vi "9_3_2_8 Control_Signal_Test_Set SW3 OFF_R.vi"(11 "VariantIn":variant caption="Test Config Cluster Variant In") -> (0 "System Error Out":errorcluster, 3 "variantOut":variant caption="Test Config Cluster V ariant Out")   [LabVIEW 2020]
uses:
  <vilib>/Utility/miscctls.llb/LVRowAndColumnTypeDef.ctl
  <userlib>/_ATMF/Tools/Control/__TEST__SEQ__VARIABLES__.ctl
  <userlib>/_ATMF/Tools/Control/__STEP__DATA__.ctl
  <userlib>/_ATMF/Tools/Control/__STEP__DATA__TYPE__.ctl
  <userlib>/_ATMF/Tools/Control/__STEP__DATA__STATUS__TYPE__.ctl
  <userlib>/_ATMF/Tools/Control/__TEST__SEQ__CONFIG__CLUSTER__.ctl
  <userlib>/_ATMF/Control_Typedef/__TEST__STEP__VAR__UI__EXEC__MODE__.ctl
  <vilib>/Utility/miscctls.llb/LVBoundsTypeDef.ctl
  <vilib>/Utility/miscctls.llb/LVPositionTypeDef.ctl
  <userlib>/_ATMF/Tools/Control/__TABLE__ACTION__.ctl
  subvi/DM3058 Function Choose.ctl
  subvi/DCDC_Command.ctl
  70cdd13f-c836-49cb-97c4-706e2b611909.vi
  259f7c0d-0f00-4e2c-849c-bbf7e935248c.vi
  <vilib>/Utility/file.llb/Write Delimited Spreadsheet (string).vi
  <vilib>/Utility/file.llb/Read Delimited Spreadsheet (string).vi
  <userlib>/_ATMF/Tools/SubVIs/SubPalette_Update_Sequencer_Variable/SEQ.Update_Seq_Var_Module.Action.vi
  <userlib>/_ATMF/Tools/SubVIs/SubPalette_Update_Sequencer_Variable/SEQ.Update_Seq_Var_Module.Pass_Fail_Test.vi
  <userlib>/_ATMF/Tools/SubVIs/SubPalette_Update_Sequencer_Variable/Set_Max_Min/SEQ.Update_Seq_Var_Module.Set_Max_Min.vi
  <userlib>/_ATMF/Tools/SubVIs/SubPalette_Update_Sequencer_Variable/SEQ.Update_Seq_Var_Module.Numericl_Test.vi
  <vilib>/Comparison/Equal/Equal Functor/Equal Functor.lvclass
  <vilib>/addons/_JKI.lib/Serialization/JSON/JKI JSON Serialization.lvlib
  a62a6993-2855-4a98-a1d5-fd509ee8ed4e.vi
  fb335dba-24a3-4358-828e-e0ecb5c05990.vi
panel:
  in  "Instrument Serial":T1
  out "Cell Position":T2
  in  "stepsRing":u16(ring) items=["Next", "End", "--------------", "init", "Measure VPS1", "Measure VPS2", "Measure VPS3"]
  in  "exitButton":bool
  in  "saveButton":bool
  in  "runButton":bool
  in  "currentRetest":u8
  in  "totalSeqIndex":i32
  in  "currenIndex":i32
  in  "seqData[](Process)":string[][](array[string])
  in  "disMsg":refnum<vi>
  in  "seqData[](Original)":string[][](array[string])
  in  "Tab Control":enum32{"Sequence", "Input", "Output"}(tab)
  in  "stepName":string
  in  "Sequence List":i32[](listbox)=[0]
  in  "seqFilePath":path caption="Sequence File Path :"
  in  "userDef":T3={"VSP1 Min"=13.0, "VSP1 Max"=11.0, "VSP2 Min"=13.0, "VSP3 Max"=11.0, "VSP3 Min"=13.0, "VSP2 Max"=11.0, "L1 Min"=1.164, "L1 Max"=1.236, "L3 Min"=1.164, "L3 Max"=1.236, "D5 Min"=1.164, "D5 Max"=1.236, "D6 Min"=1.164, "D6 Max"=1.236, "D3 Min"=0.873, "D3 Max"=0.927, "D8 Min"=1.164, "D8 Max"=1.236, "APOS Max "=0.5, "ANEG Max"=-0.5, "DPOS Max"=0.5, "APOS Min"=0.5, "ANEG Min"=-0.5, "DPOS Min"=0.5} caption="User Input ( Save by Run Ctrl+R and click \"Save\" button  )"
  in  "varFilePath":path caption="Variable File Path :"
  in  "criteriaINI":path caption="Criteria(.ini) Path :"
  in  "displayMsg":string caption="Display Message"
  in  "testTable":i32(listbox)=-1 caption="Connectivity Test"
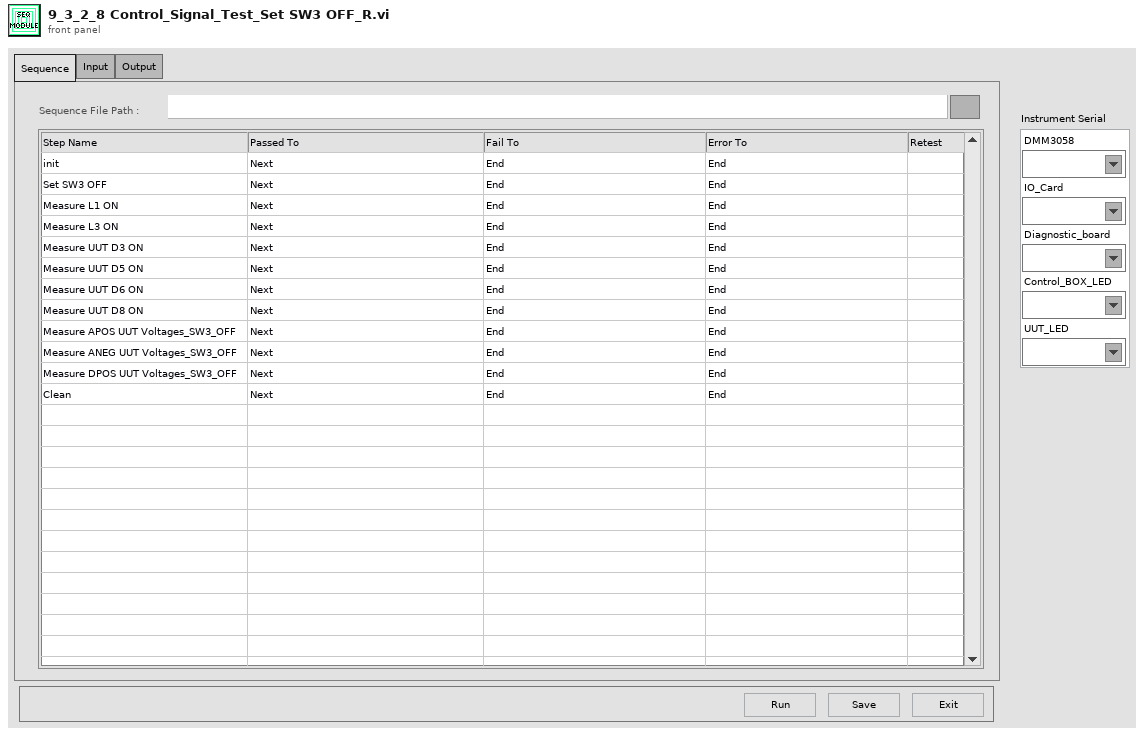
[diagram p1: front panel]
types:
  T1 = cluster{"DMM3058":refnum<visa-resource-name>, "IO_Card":refnum<visa-resource-name>, "Diagnostic_board":refnum<visa-resource-name>, "Control_BOX_LED":refnum<visa-resource-name>, "UUT_LED":refnum<visa-resource-name>}
  T2 = typedef "LVRowAndColumnTypeDef.ctl" = cluster{"Row":i32, "Column":i32}
  T3 = cluster{"VSP1 Min":dbl, "VSP1 Max":dbl, "VSP2 Min":dbl, "VSP3 Max":dbl, "VSP3 Min":dbl, "VSP2 Max":dbl, "L1 Min":dbl, "L1 Max":dbl, "L3 Min":dbl, "L3 Max":dbl, "D5 Min":dbl, "D5 Max":dbl, "D6 Min":dbl, "D6 Max":dbl, "D3 Min":dbl, "D3 Max":dbl, "D8 Min":dbl, "D8 Max":dbl, "APOS Max ":dbl, "ANEG Max":dbl, "DPOS Max":dbl, "APOS Min":dbl, "ANEG Min":dbl, "DPOS Min":dbl}
  T4 = typedef "__TEST__SEQ__VARIABLES__.ctl" = cluster{"stepData":T5, "testConfigCluster":T8}
  T5 = typedef "__STEP__DATA__.ctl" = cluster{"stepType":T6, "stepName":string, "description":string, "min":string, "measure":string, "max":string, "unit":string, "statusType":T7, "runMode":enum16{"Normal", "Skip"}, "viPath":path, "uutError":errorcluster, "passTo":string, "failTo":string, "errorTo":string, "parameter":string, "value":variant, "startTime":timestamp, "intervalLoop":u8, "retest":u8}
  T6 = typedef "__STEP__DATA__TYPE__.ctl" = enum16{"Action", "Pass/Fail Test", "Numeric Limit Test", "String Value Test"}
  T7 = typedef "__STEP__DATA__STATUS__TYPE__.ctl" = enum16{"DONE", "PASS", "FAIL", "ERROR", "SKIPPED"}
  T8 = typedef "__TEST__SEQ__CONFIG__CLUSTER__.ctl" = cluster{"slotIndex":u8, "execMode":T9, "mainConfigFile":path, "criteriaINI":path, "totalResult":bool, "stopIfFail":bool, "userControls":cluster{"dialog":refnum<vi>, "testTable":refnum<vi>, "stopButton":refnum<vi>, "statusBox":refnum<vi>}, "testedResult":enum16{"DONE", "PASS", "FAIL", "ERROR", "SKIPPED"}, "timeStamp":cluster{"Start":timestamp, "End":timestamp}, "repeatNum":u8, "uutInfo":cluster{"s/n":string, "p/n":string, "productRev":string}, "sysLanguage":enum16{"English", "Chinese", "Thai"}, "numOfSocket#":u8, "testRef":string, "testInfo":cluster{"testTime":string, "userID":string, "stationName":string, "testerID":string, "hwVer":string, "swVer":string, "fixtureID":string}}
  T9 = typedef "__TEST__STEP__VAR__UI__EXEC__MODE__.ctl" = enum16{"Run", "Debug", "Edit", "Open VI"}
  T10 = enum16{"open", "replace", "create", "open or create", "replace or create", "replace or create with confirmation"}
  T11 = typedef "LVPositionTypeDef.ctl" = cluster{"Left":i32, "Top":i32}
  T12 = typedef "LVBoundsTypeDef.ctl" = cluster{"Width":u32, "Height":u32}
  T13 = enum32{"Bad", "Idle", "Run top level", "Running"}
  T14 = typedef "__TABLE__ACTION__.ctl" = enum16{"Initial", "Append", "Clear", "Header"}
  T15 = enum16{"StepName", "PassTo", "FailTo", "ErrorTo", "Re-test"}
  T16 = enum16{"StepName", "PassTo", "FailTo", "ErrorTo"}
  T17 = cluster{"Reset (True)":bool, "ID Query (True)":bool, "Auto Range (T:Enable)":bool, "Function (0: DC Volts)":u16, "Range Select":enum16{"200mV", "2V", "20V", "200V", "1000V"}, "Absolute Resolution (0: 5.5 Rate:Slow)":u16}
  T18 = typedef "DM3058 Function Choose.ctl" = enum16{"Close", "Measure", "Config", "Init"}
  T19 = typedef "DCDC_Command.ctl" = enum16{"Reset", "APOS_SENSE", "ANEG_SENSE", "DPOS_SENSE", "FCT_SW1", "FCT_SW2", "FCT_SW3", "ANEG_LOAD", "APOS_LOAD", "DPOS_LOAD", "Short ANEG", "Short APOS", "Short DPOS", "meas_PSU_1_12V", "meas_PSU_2_12V", "meas_PSU_3_12V", "meas_UUT_APOS_voltage", "meas_UUT_ANEG_voltage", "meas_UUT_DPOS_voltage", "meas_LOAD_APOS_voltage", "meas_LOAD_ANEG_voltage", "meas_LOAD_DPOS_voltage", "UUT_FCT_power_SW", "Burn_in_FAN_SW", "FCT_FAN_SW", "FCT_24V_SW", "USB_Reset", "DMM_SW"}
  T20 = typedef "LVPoint32TypeDef.ctl" = cluster{"Horizontal":i32, "Vertical":i32}
  T21 = typedef "LVFontTypeDef.ctl" = cluster{"Font Name":string, "Size":u16, "Bold":bool, "Italic":bool, "Underline":bool, "Strikeout":bool, "Color":u32}
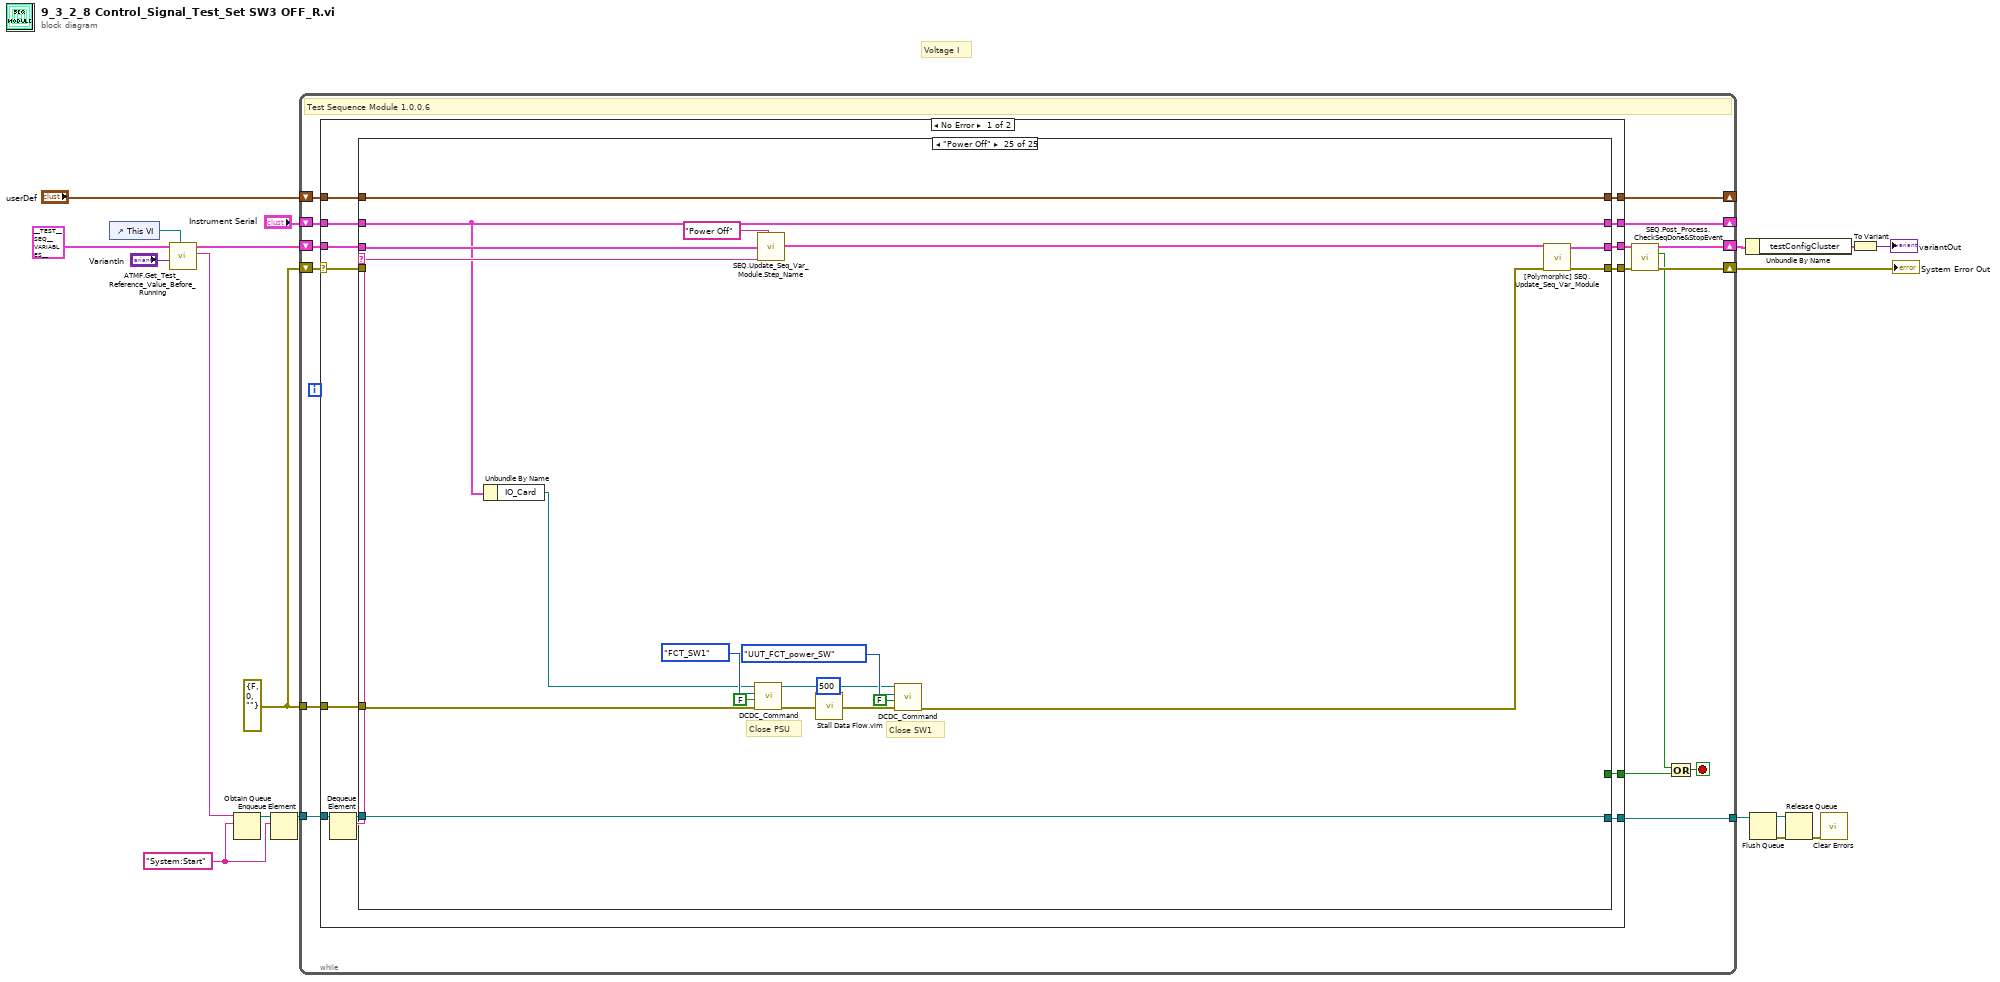
[diagram p0: block diagram]
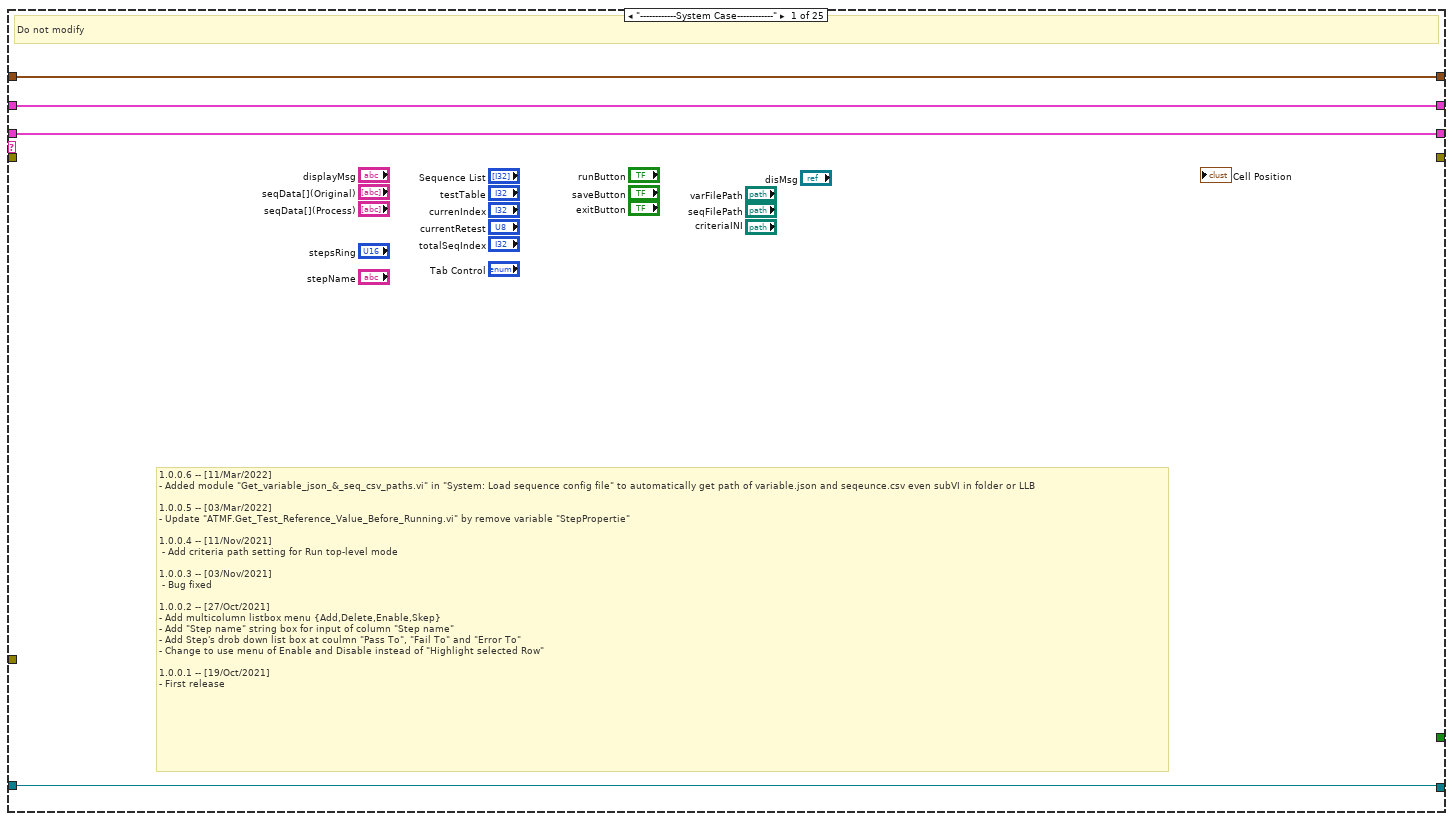
[diagram p2: hidden frame]
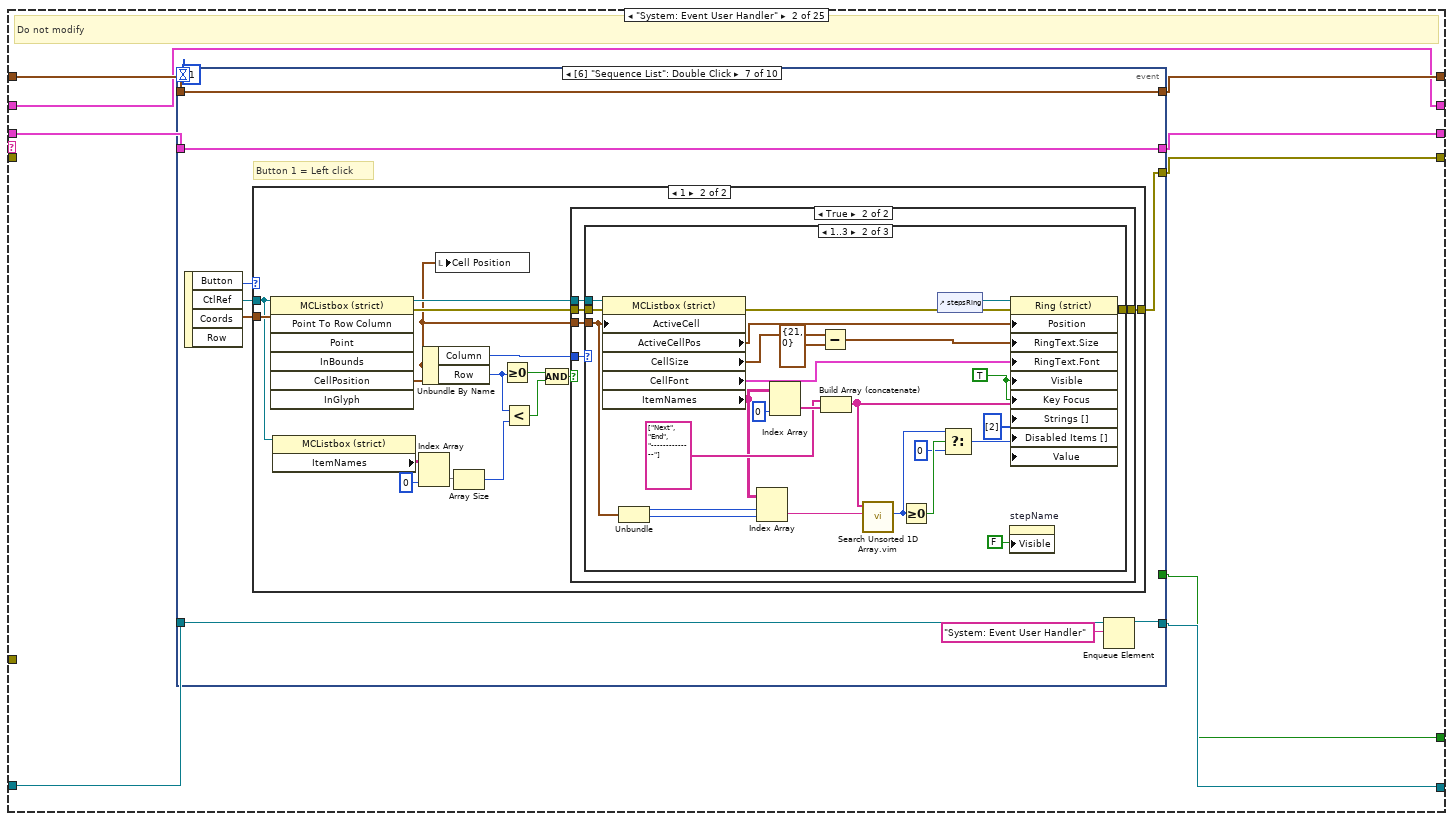
[diagram p3: hidden frame]
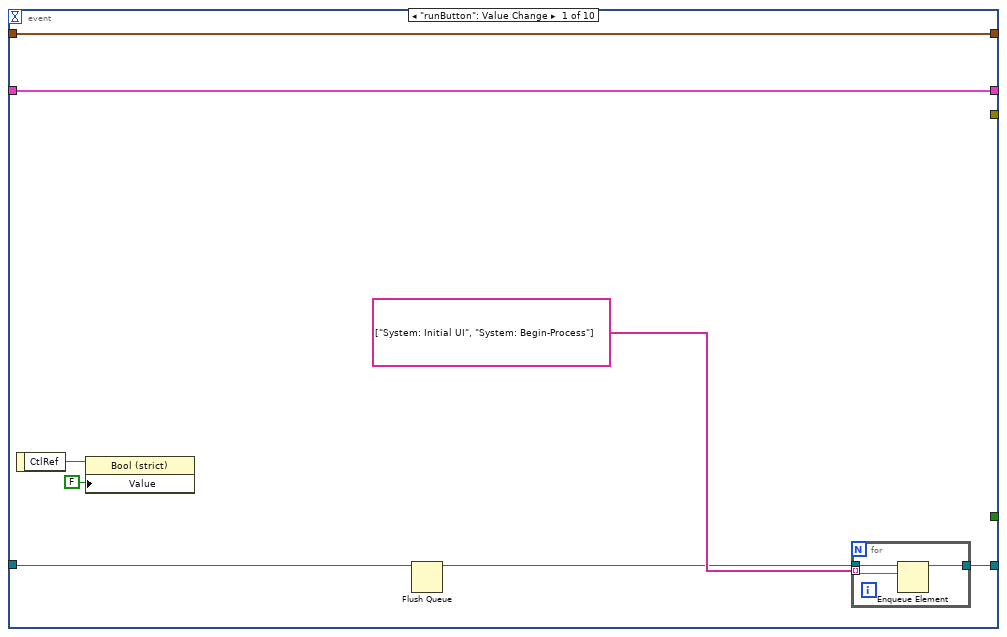
[diagram p4: hidden frame]
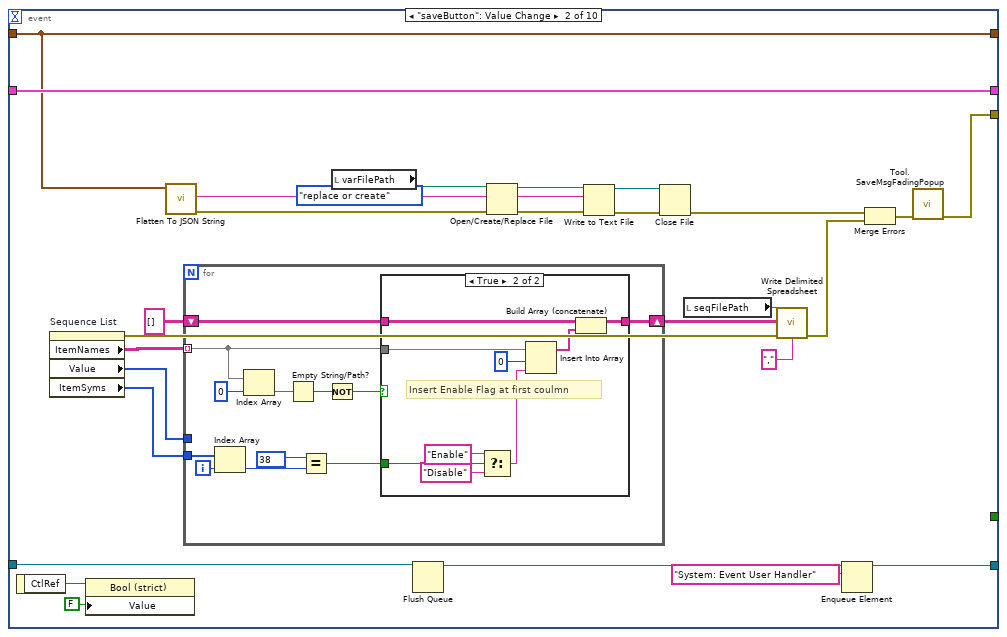
[diagram p5: hidden frame]
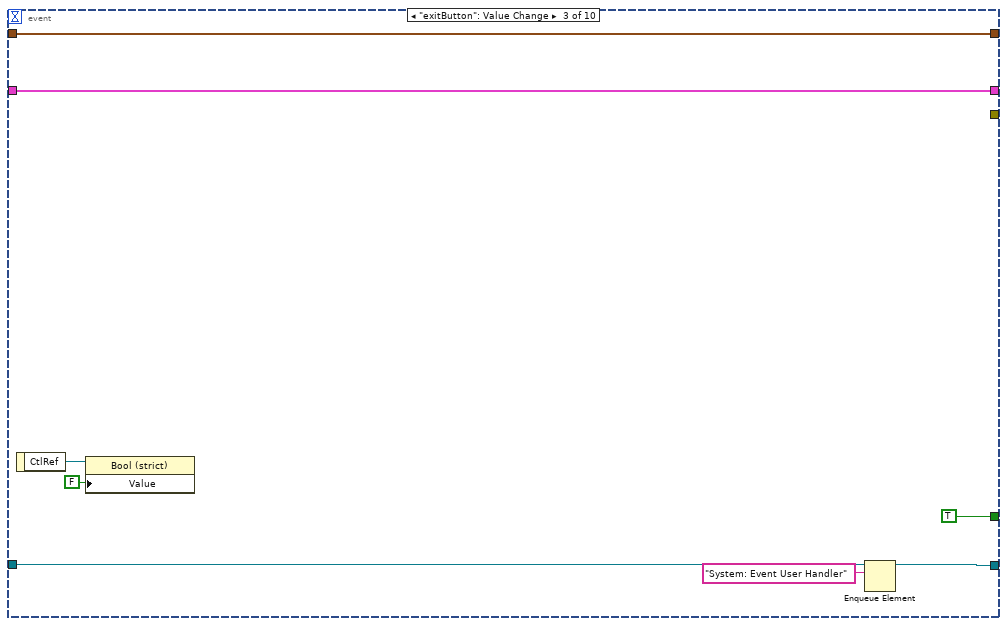
[diagram p7: hidden frame]
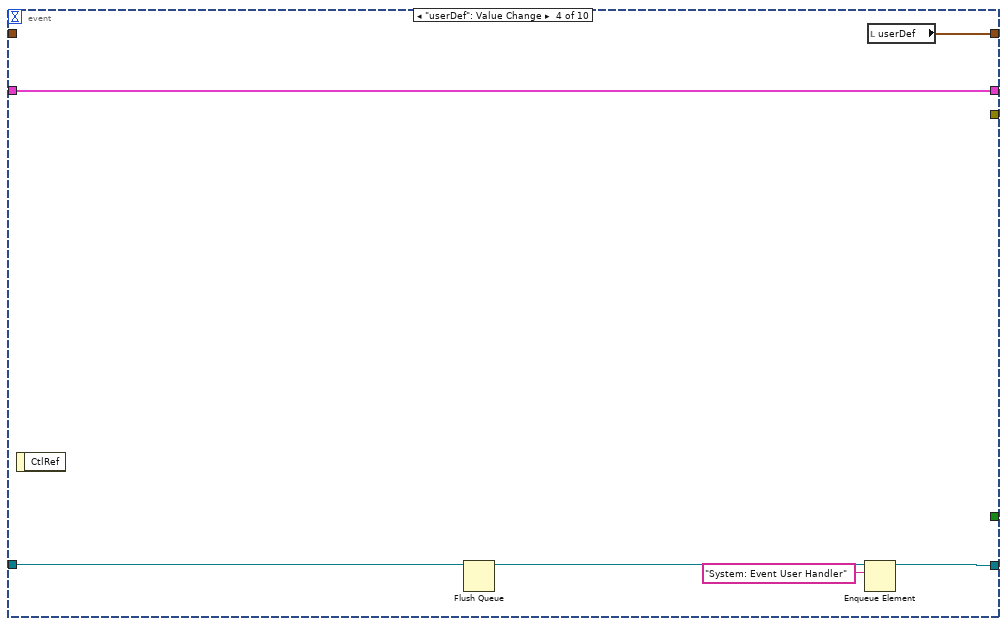
[diagram p8: hidden frame]
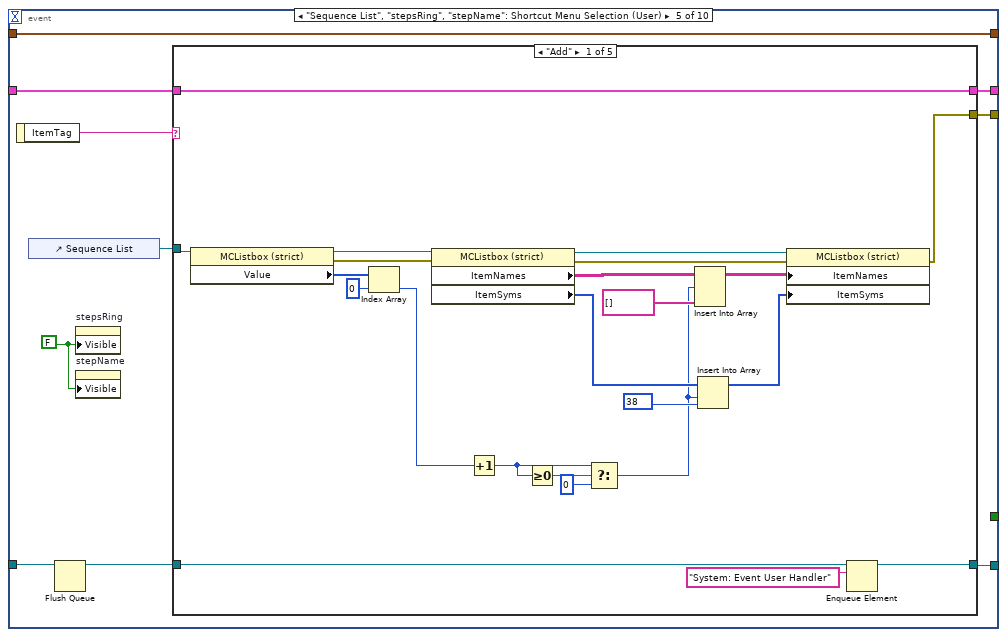
[diagram p9: hidden frame]
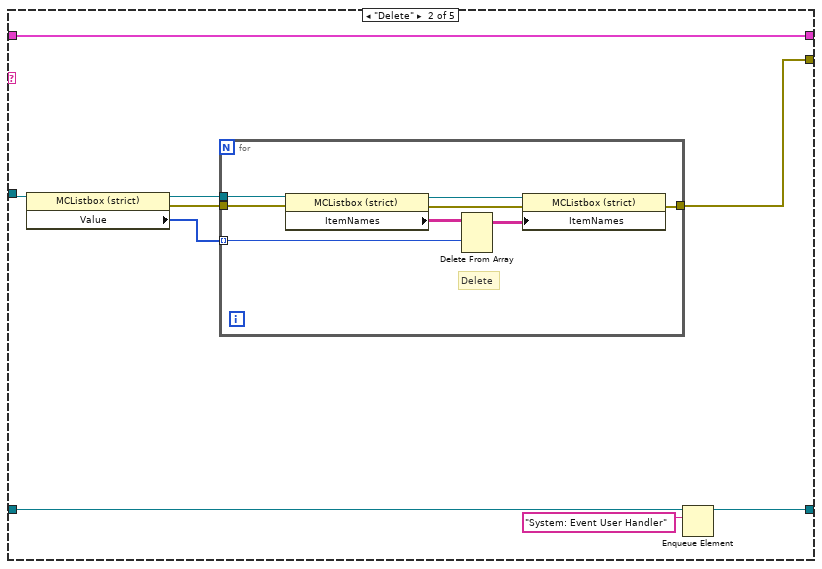
[diagram p10: hidden frame]
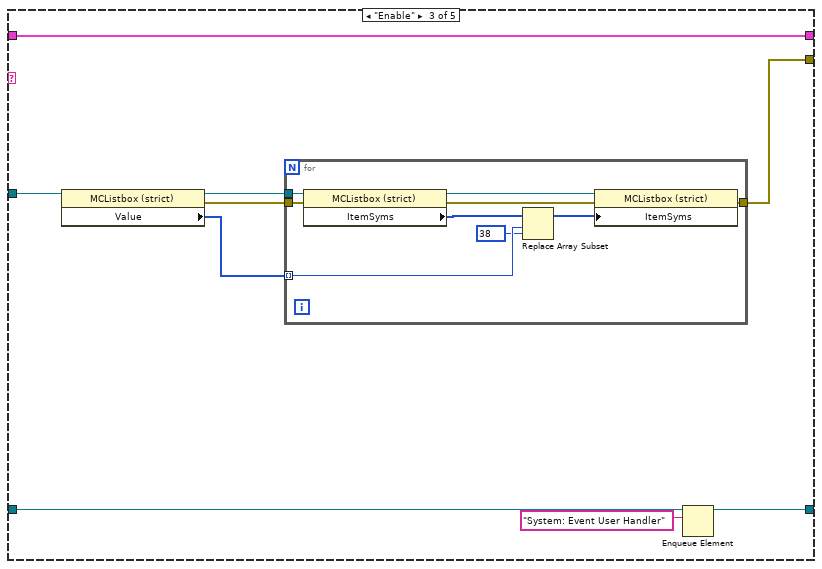
[diagram p11: hidden frame]
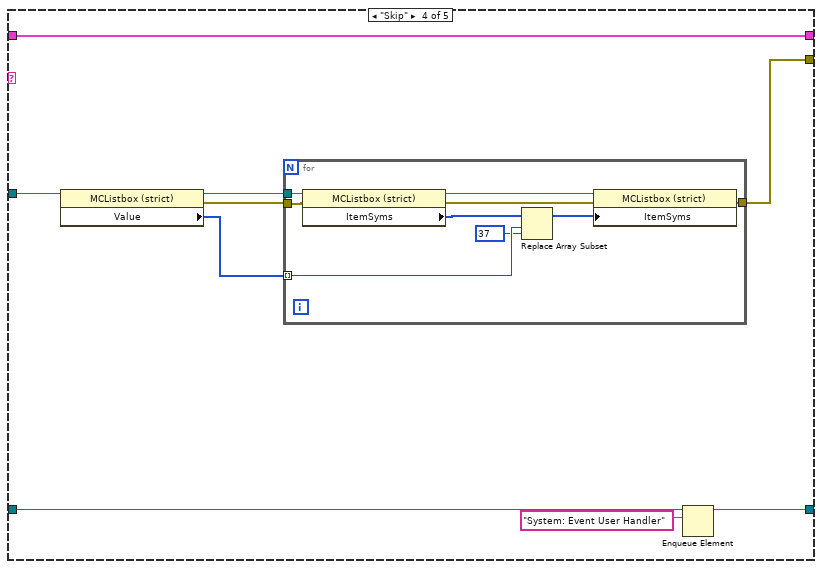
[diagram p12: hidden frame]
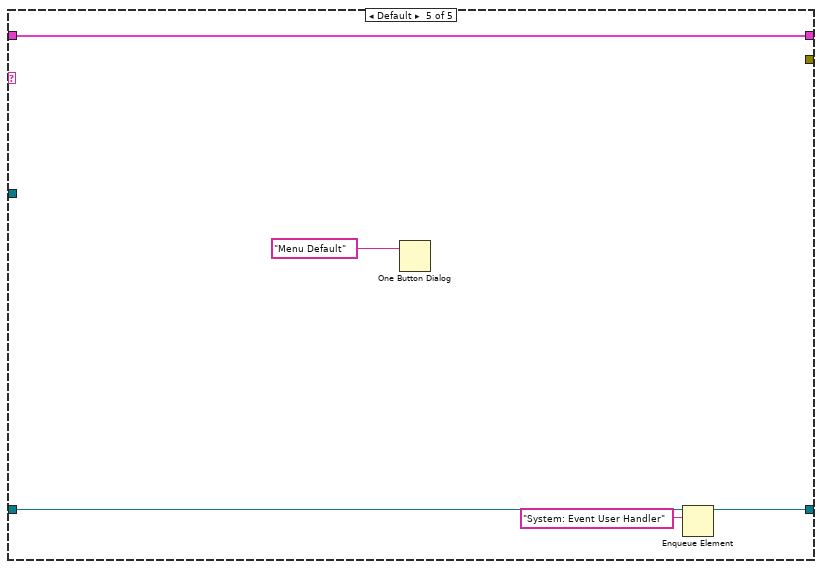
[diagram p13: hidden frame]
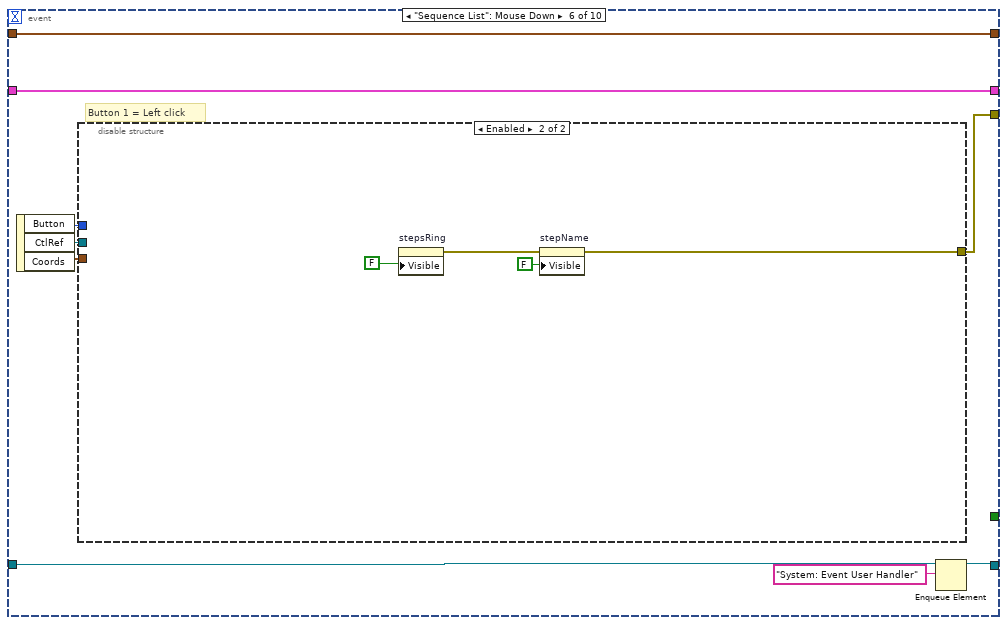
[diagram p14: hidden frame]
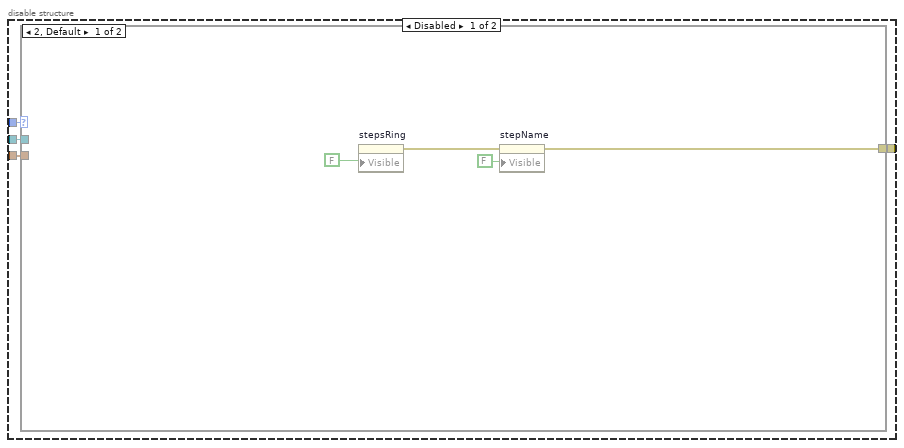
[diagram p15: hidden frame]
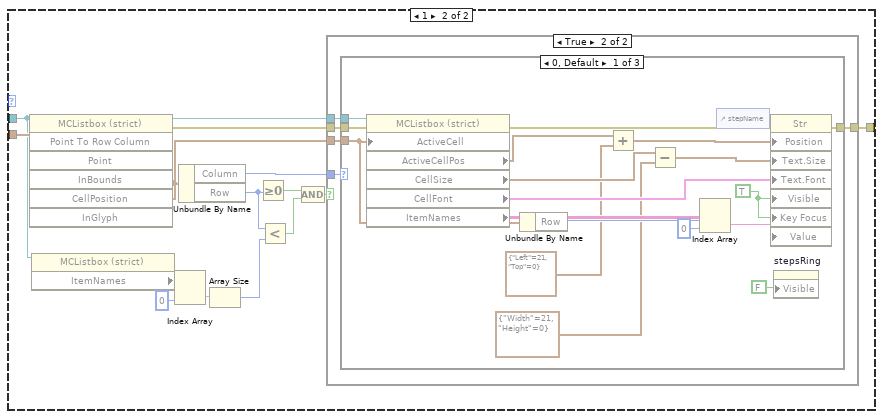
[diagram p16: hidden frame]
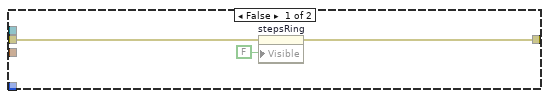
[diagram p17: hidden frame]
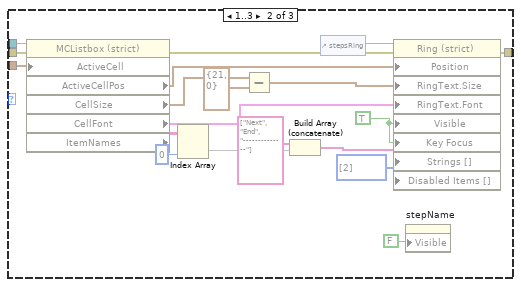
[diagram p18: hidden frame]
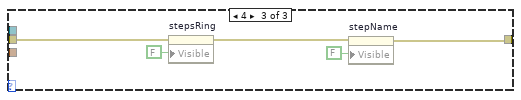
[diagram p19: hidden frame]
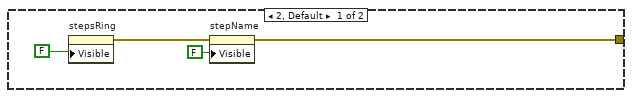
[diagram p20: hidden frame]
diagram:
  w2 = errorcluster {"status"=FALSE, "code"=0, "source"=""} ("UUT Error In")
  w14 = "System:Start"
  # "Voltage I"
  n1 = control-ref of="This VI"() -> (w6:refnum<vi>)
  n2 = call <userlib>:"ATMF.Get_Test_Reference_Value_Before_Running.vi"("viRef"=w6, "Variant"="VariantIn", "seqDataIn"=T4 {"stepData"={"stepType"=enum."Action", "stepName"="", "description"="", "min"="", "measure"="", "max"="", "unit"="", "statusType"=enum."DONE", "runMode"=enum."Normal", "viPath"=path "", "uutError"={"status"=FALSE, "code"=0, "source"=""}, "passTo"="", "failTo"="", "errorTo"="", "parameter"="", "value"=variant(string[][] []), "startTime"=timestamp(0 s since 1904-01-01), "intervalLoop"=1, "retest"=0}, "testConfigCluster"={"slotIndex"=0, "execMode"=enum."Run", "mainConfigFile"=path "", "criteriaINI"=path "", "totalResult"=FALSE, "stopIfFail"=FALSE, "userControls"={"dialog"=refnum, "testTable"=refnum, "stopButton"=refnum, "statusBox"=refnum}, "testedResult"=enum."DONE", "timeStamp"={"Start"=timestamp(0 s since 1904-01-01), "End"=timestamp(0 s since 1904-01-01)}, "repeatNum"=1, "uutInfo"={"s/n"="", "p/n"="", "productRev"=""}, "sysLanguage"=enum."English", "numOfSocket#"=1, "testRef"="", "testInfo"={"testTime"="", "userID"="", "stationName"="", "testerID"="", "hwVer"="", "swVer"="", "fixtureID"=""}}} ("localVar")) -> ("testRef#"=w9:string, "seqDataOut"=w7:T4)  [unwired: 6 in, 1 out]
  n3 = Obtain Queue(name (unnamed)=w9, element data type=w14) -> (queue out=w19:refnum<queue>)  [unwired: 3 in, 2 out]
  n4 = Enqueue Element(queue=w19, element=w14) -> (queue out=w17:refnum<queue>)  [unwired: 2 in, 2 out]
  n5 = while {
    shift-right: [w25] -> w11
    shift-left: w2 -> [w35]
    shift-right: [w27] -> w5
    shift-left: w7 -> [w34]
    tunnel: w17 -> [w33]
    tunnel: [w32] -> w16
    tunnel: w2 -> [w30]
    shift-right: [w29] -> _
    shift-left: "userDef" -> [w31]
    shift-right: [w21] -> _
    shift-left: "Instrument Serial" -> [w20]
    stop <- w22 stop-if-true
    # "Test Sequence Module 1.0.0.6"
    n6 = case shown="No Error" w35 {
      selector: w35 -> [w47 w1153]
      tunnel: [w46 w1153] -> w26
      tunnel: w34 -> [w49 w1160]
      tunnel: [w48 w1160] -> w28
      tunnel: [w45 TRUE] -> w23
      tunnel: [w42 w1158] -> w32
      tunnel: w33 -> [w41 w1155]
      tunnel: w31 -> [w39 w1154]
      tunnel: w30 -> [w40 _]
      tunnel: [w38 w1154] -> w29
      tunnel: [w37 w1152] -> w21
      tunnel: w20 -> [w36 w1152]
      frame No Error {
        n7 = Dequeue Element(queue=w41) -> (queue out=w43:refnum<queue>, element=w44:string)  [unwired: 2 in, 2 out]
        n8 = case shown="\"Power Off\"" w44 {
          selector: w44 -> [_ _ _ _ _ _ _ _ _ _ _ w763 _ w776 w820 w843 w866 w890 w912 w935 w959 w981 w1036 w1089 w1149]
          tunnel: w49 -> [w52 w60 w438 w472 w484 w535 w622 w638 w683 w707 w740 w767 w770 w814 w821 w855 w878 w901 w924 w947 w970 w996 w1050 w1104 w1148]
          tunnel: [w52 w59 w440 w475 w493 w535 w622 w640 w682 w715 w743 w767 w770 w813 w818 w854 w877 w900 w923 w946 w969 w993 w1047 w1101 w1144] -> w48
          tunnel: w47 -> [_ _ _ _ _ _ _ _ _ _ _ _ _ w775 w819 w844 w871 w889 w917 w940 w958 w982 w1035 w1091 _]
          tunnel: [_ w55 _ _ w494 w533 _ _ _ _ _ w759 _ w812 w817 w853 w876 w899 w922 w945 w968 w994 w1048 w1102 w1145] -> w46
          tunnel: [_ w56 _ _ _ _ _ _ _ _ w746 TRUE _ _ _ _ _ _ _ _ _ _ _ _ _] -> w45
          tunnel: w43 -> [w51 w63 w450 w473 w491 w536 w628 w642 w681 w714 w742 w765 w769 w811 _ w852 w875 w898 w921 w944 w967 w997 w1051 w1105 w1146]
          tunnel: [w51 w58 w449 w473 w490 w536 w627 w641 w680 w713 w741 w765 w769 w811 _ w852 w875 w898 w921 w944 w967 w997 w1051 w1105 w1146] -> w42
          tunnel: w40 -> [_ _ _ _ _ _ _ _ _ _ _ _ _ w790 w824 w842 w863 w885 w909 w931 w955 w990 w1044 w1100 w1141]
          tunnel: w39 -> [w53 w62 w442 w474 w495 w532 w617 w639 w685 w716 w745 w764 w771 w809 w823 w851 w874 w897 w920 w943 w966 w988 w1042 w1096 w1147]
          tunnel: [w53 w61 w441 w474 w495 w531 w617 w639 w685 w716 w744 w764 w771 w809 w823 w851 w874 w897 w920 w943 w966 w988 w1042 w1096 w1147] -> w38
          tunnel: [w50 w54 w436 w470 w483 w526 w616 w629 w679 w705 w738 w757 w768 w781 w822 w849 w872 w895 w918 w941 w964 w992 w1043 w1098 w1134] -> w37
          tunnel: w36 -> [w50 w54 w436 w470 w483 w526 w616 w629 w679 w705 w738 w757 w768 w808 w822 w849 w872 w895 w918 w941 w964 w992 w1043 w1098 w1134]
          frame "------------System Case------------" {
            # "1.0.0.6 -- [11/Mar/2022]\n- Added module \"Get_variable_json_&_seq_csv_paths.vi\" in \"System: Load sequence config file\" to automatically get path of variable.json and seqeunce.csv even subVI in folder or LLB\n\n1.0.0.5 -- [03/Mar/2022]\n- Update \"ATMF.Get_Test_Reference_Value_Before_Running.vi\" by remove variable \"StepPropertie\"\n\n1.0.0.4 -- [11/Nov/2021]\n - Add criteria path setting for Run top-level mode\n\n1.0.0.3 -- [03/Nov/2021]\n - Bug fixed \n\n1.0.0.2 -- [27/Oct/2021]\n- Add multicolumn listbox menu {Add,Delete,Enable,Skep}\n- Add \"Step name\" string box for input of column \"Step name\"\n- Add Step's drob down list box at coulmn \"Pass To\", \"Fail To\" and \"Error To\"\n- Change to use menu of Enable and Disable instead of \"Highlight selected Row\"\n\n1.0.0.1 -- [19/Oct/2021]\n- First release"
            # "Do not modify"
          }
          frame "System: Event User Handler" {
            # "Do not modify"
            n9 = event shown="[6] \"Sequence List\": Double Click" {
              selector: _ -> [_ _ _ _ _ _ _ _ _ _]
              dyn-events: _ -> [_ _ _ _ _ _ _ _ _ _]
              timeout: -1 -> [_ _ _ _ _ _ _ _ _ _]
              tunnel: w63 -> [w64 w86 w126 w133 w142 w236 w323 w404 w424 w433]
              tunnel: w62 -> [w71 w99 w132 _ w147 w238 w325 w415 w432 w435]
              tunnel: [w71 w99 w132 w135 w147 w238 w325 w415 w432 w435] -> w61
              tunnel: w60 -> [w70 w102 w131 w138 w145 w237 w324 w414 w431 w434]
              tunnel: [w70 w102 w131 w138 w146 w237 w324 w414 w431 w434] -> w59
              tunnel: [w69 w89 w127 w137 w148 w235 w322 w405 w425 w433] -> w58
              tunnel: [_ _ TRUE _ _ _ _ _ _ _] -> w56
              tunnel: [_ w97 _ _ w141 w231 w318 w411 w428 _] -> w55
              event "runButton": Value Change {
                n10 = event-data() -> ("CtlRef"=w68:refnum<vi>)  [unwired: 1 in]
                n11 = property class="Bool (strict)"(reference=w68, "Value"=FALSE) -> ()  [unwired: 1 in, 2 out]
                n12 = Flush Queue(queue=w64) -> (queue out=w65:refnum<queue>)  [unwired: 1 in, 2 out]
                n13 = for {
                  tunnel: w65 -> [w74]
                  tunnel: [w73] -> w69
                  tunnel: string[] ["System: Initial UI", "System: Begin-Process"] -> [w72] mode=indexing
                  n14 = Enqueue Element(queue=w74, element=w72) -> (queue out=w73:refnum<queue>)  [unwired: 2 in, 2 out]
                }
              }
              event "saveButton": Value Change {
                n15 = event-data() -> ("CtlRef"=w101:refnum<vi>)  [unwired: 1 in]
                n16 = property on="Sequence List" class="MCListbox (strict)"() -> (error out=w85:errorcluster, "ItemNames"=w81:string[][], "Value"=w82:i32[], "ItemSyms"=w75:i32[])  [unwired: 2 in, 1 out]
                n17 = property class="Bool (strict)"(reference=w101, "Value"=FALSE) -> ()  [unwired: 1 in, 2 out]
                n18 = call <vilib>:"Flatten To JSON String.vi"("Variant"=w99) -> ("error out"=w98:errorcluster, "JSON String"=w91:string)  [unwired: 9 in]
                n19 = for {
                  tunnel: w82 -> [_]
                  tunnel: w81 -> [w112] mode=indexing
                  shift-right: [w108] -> w79
                  shift-left: string[][] [] -> [w109]
                  tunnel: w75 -> [w107]
                  i -> [w106]
                  n20 = Index Array(array=w107, index=w106) -> (element=w105:i32)
                  n21 = Index Array(array=w112, index=0) -> (element=w110:string)
                  n22 = Empty String/Path?(string/path=w110) -> (empty?=w114:bool)
                  n23 = Equal?(x=38, y=w105) -> (x = y?=w103:bool)
                  n24 = Not(x=w114) -> (.not. x?=w113:bool)
                  n25 = case shown="True" w113 {
                    tunnel: w112 -> [_ w124]
                    tunnel: w109 -> [w115 w120]
                    tunnel: [w115 w119] -> w108
                    tunnel: w103 -> [_ w116]
                    frame False {
                    }
                    frame True {
                      # "Insert Enable Flag at first coulmn"
                      n26 = Select(t="Enable", s=w116, f="Disable") -> (s? t:f=w121:string)
                      n27 = Insert Into Array(array=w124, index=0, new element=w121) -> (w118:string[])
                      n28 = Build Array (concatenate)(w120, w118) -> (w119:string[][])
                    }
                  }
                }
                n29 = local read "varFilePath"() -> (w92:path)
                n30 = Flush Queue(queue=w86) -> (queue out=w87:refnum<queue>)  [unwired: 1 in, 2 out]
                n31 = Open/Create/Replace File(file path (use dialog)=w92, error in=w98, operation (0:open)=T10."replace or create") -> (refnum out=w94:refnum<file>, error out=w96:errorcluster)  [unwired: 3 in, 1 out]
                n32 = Write to Text File(file (use dialog)=w94, text=w91, error in=w96) -> (refnum out=w93:refnum<file>, error out=w95:errorcluster)  [unwired: 1 in, 1 out]
                n33 = Close File(refnum=w93, error in=w95) -> (error out=w77:errorcluster)  [unwired: 1 out]
                n34 = local read "seqFilePath"() -> (w83:path)
                n35 = call-poly <vilib>:"Write Delimited Spreadsheet.vi"("file path (dialog if empty)"=w83, "2D data"=w79, "error in (no error)"=w85, "delimiter (\\t)"="," ("delimiter (\\t)")) -> ("error out"=w78:errorcluster)  [unwired: 10 in, 1 out]
                n36 = Enqueue Element(queue=w87, element="System: Event User Handler") -> (queue out=w89:refnum<queue>)  [unwired: 2 in, 2 out]
                n37 = Merge Errors(w77, w78) -> (w76:errorcluster)
                n38 = call <userlib>:"Tool.SaveMsgFadingPopup.vi"("error in"=w76) -> ("error out"=w97:errorcluster)  [unwired: 10 in]
              }
              event "exitButton": Value Change {
                n39 = event-data() -> ("CtlRef"=w130:refnum<vi>)  [unwired: 1 in]
                n40 = property class="Bool (strict)"(reference=w130, "Value"=FALSE) -> ()  [unwired: 1 in, 2 out]
                n41 = Enqueue Element(queue=w126, element="System: Event User Handler") -> (queue out=w127:refnum<queue>)  [unwired: 2 in, 2 out]
              }
              event "userDef": Value Change {
                n42 = event-data() -> ()  [unwired: 1 in, 1 out]
                n43 = Flush Queue(queue=w133) -> (queue out=w134:refnum<queue>)  [unwired: 1 in, 2 out]
                n44 = Enqueue Element(queue=w134, element="System: Event User Handler") -> (queue out=w137:refnum<queue>)  [unwired: 2 in, 2 out]
                n45 = local read "userDef"() -> (w135:T3)
              }
              event "Sequence List", "stepsRing", "stepName": Shortcut Menu Selection (User) {
                w139 = FALSE
                n46 = event-data() -> ("ItemTag"=w144:string)  [unwired: 1 in]
                n47 = control-ref of="Sequence List"() -> (w140:refnum<vi>)
                n48 = Flush Queue(queue=w142) -> (queue out=w143:refnum<queue>)  [unwired: 1 in, 2 out]
                n49 = property on="stepsRing" class="Ring (strict)"("Visible"=w139) -> ()  [unwired: 2 in, 2 out]
                n50 = property on="stepName" class="Str"("Visible"=w139) -> ()  [unwired: 2 in, 2 out]
                n51 = case shown="\"Add\"" w144 {
                  tunnel: [w171 w180 w197 w215 w229] -> w148
                  tunnel: w143 -> [w169 w178 w195 w213 w227]
                  tunnel: [w168 w177 w194 w212 w226] -> w146
                  tunnel: w145 -> [w168 w177 w194 w212 w226]
                  tunnel: w140 -> [w149 w173 w193 w211 _]
                  tunnel: [w161 w174 w189 w207 _] -> w141
                  frame "Add" {
                    n52 = property class="MCListbox (strict)"(reference=w149) -> (reference out=w165:refnum<vi>, error out=w164:errorcluster, "Value"=w167:i32[])  [unwired: 1 in]
                    n53 = Index Array(array=w167, index=0) -> (element=w152:i32)
                    n54 = property class="MCListbox (strict)"(reference=w165, error in=w164) -> (reference out=w163:refnum<vi>, error out=w162:errorcluster, "ItemNames"=w160:string[][], "ItemSyms"=w157:i32[])
                    n55 = Increment(x=w152) -> (x+1=w154:i32)
                    n56 = Greater Or Equal To 0?(x=w154) -> (x >= 0?=w153:bool)
                    n57 = Select(t=w154, s=w153, f=0) -> (s? t:f=w151:i32)
                    n58 = Insert Into Array(array=w160, index (row)=w151, new element=string[] [] ("new element/subarray")) -> (w159:string[][])  [unwired: 1 in]
                    n59 = Insert Into Array(array=w157, index=w151, new element=38) -> (w155:i32[])
                    n60 = property class="MCListbox (strict)"(reference=w163, error in=w162, "ItemNames"=w159, "ItemSyms"=w155) -> (error out=w161:errorcluster)  [unwired: 1 out]
                    n61 = Enqueue Element(queue=w169, element="System: Event User Handler") -> (queue out=w171:refnum<queue>)  [unwired: 2 in, 2 out]
                  }
                  frame "Delete" {
                    n62 = property class="MCListbox (strict)"(reference=w173) -> (reference out=w176:refnum<vi>, error out=w175:errorcluster, "Value"=w172:i32[])  [unwired: 1 in]
                    n63 = for {
                      tunnel: w176 -> [w188]
                      tunnel: w175 -> [w187]
                      tunnel: [w184] -> w174
                      tunnel: w172 -> [w182] mode=indexing
                      # "Delete"
                      n64 = property class="MCListbox (strict)"(reference=w188, error in=w187) -> (reference out=w186:refnum<vi>, error out=w185:errorcluster, "ItemNames"=w183:string[][])
                      n65 = Delete From Array(array=w183, index (row)=w182) -> (array with subset deleted=w181:string[][])  [unwired: 2 in, 1 out]
                      n66 = property class="MCListbox (strict)"(reference=w186, error in=w185, "ItemNames"=w181) -> (error out=w184:errorcluster)  [unwired: 1 out]
                    }
                    n67 = Enqueue Element(queue=w178, element="System: Event User Handler") -> (queue out=w180:refnum<queue>)  [unwired: 2 in, 2 out]
                  }
                  frame "Enable" {
                    n68 = property class="MCListbox (strict)"(reference=w193) -> (reference out=w191:refnum<vi>, error out=w190:errorcluster, "Value"=w192:i32[])  [unwired: 1 in]
                    n69 = for {
                      tunnel: w192 -> [w202] mode=indexing
                      tunnel: w191 -> [w206]
                      tunnel: w190 -> [w200]
                      tunnel: [w198] -> w189
                      n70 = property class="MCListbox (strict)"(reference=w206, error in=w200) -> (reference out=w204:refnum<vi>, error out=w199:errorcluster, "ItemSyms"=w205:i32[])
                      n71 = Replace Array Subset(array=w205, new element=38, index=w202) -> (w203:i32[])
                      n72 = property class="MCListbox (strict)"(reference=w204, error in=w199, "ItemSyms"=w203) -> (error out=w198:errorcluster)  [unwired: 1 out]
                    }
                    n73 = Enqueue Element(queue=w195, element="System: Event User Handler") -> (queue out=w197:refnum<queue>)  [unwired: 2 in, 2 out]
                  }
                  frame "Skip" {
                    n74 = property class="MCListbox (strict)"(reference=w211) -> (reference out=w209:refnum<vi>, error out=w208:errorcluster, "Value"=w210:i32[])  [unwired: 1 in]
                    n75 = for {
                      tunnel: w210 -> [w220] mode=indexing
                      tunnel: w209 -> [w224]
                      tunnel: w208 -> [w218]
                      tunnel: [w216] -> w207
                      n76 = property class="MCListbox (strict)"(reference=w224, error in=w218) -> (reference out=w222:refnum<vi>, error out=w217:errorcluster, "ItemSyms"=w223:i32[])
                      n77 = Replace Array Subset(array=w223, new element=37, index=w220) -> (w221:i32[])
                      n78 = property class="MCListbox (strict)"(reference=w222, error in=w217, "ItemSyms"=w221) -> (error out=w216:errorcluster)  [unwired: 1 out]
                    }
                    n79 = Enqueue Element(queue=w213, element="System: Event User Handler") -> (queue out=w215:refnum<queue>)  [unwired: 2 in, 2 out]
                  }
                  frame Default {
                    n80 = One Button Dialog(message="Menu Default") -> ()  [unwired: 1 in, 1 out]
                    n81 = Enqueue Element(queue=w227, element="System: Event User Handler") -> (queue out=w229:refnum<queue>)  [unwired: 2 in, 2 out]
                  }
                }
              }
              event "Sequence List": Mouse Down {
                # "Button 1 = Left click"
                n82 = event-data() -> ("Button"=w230:u16, "CtlRef"=w232:refnum<vi>, "Coords"=w233:T20)  [unwired: 1 in]
                n83 = disable-structure shown="Enabled" {
                  disable-tunnel: w233 -> [w242 _]
                  disable-tunnel: w232 -> [w241 _]
                  disable-tunnel: [w240 w313] -> w231
                  disable-tunnel: w230 -> [w239 _]
                  frame Disabled {
                    n84 = case shown="2, Default" w239 {
                      tunnel: w242 -> [_ w261]
                      tunnel: w241 -> [_ w257]
                      tunnel: [w243 w247] -> w240
                      frame 2, Default {
                        n85 = property on="stepsRing" class="Ring (strict)"("Visible"=FALSE) -> (error out=w245:errorcluster)  [unwired: 2 in, 1 out]
                        n86 = property on="stepName" class="Str"(error in=w245, "Visible"=FALSE) -> (error out=w243:errorcluster)  [unwired: 1 in, 1 out]
                      }
                      frame 1 {
                        n87 = invoke class="MCListbox (strict)" method="Point To Row Column"(reference=w257, "Point"=w261) -> (reference out=w260:refnum<vi>, error out=w259:errorcluster, "CellPosition"=w258:T2)  [unwired: 5 in, 4 out]
                        n88 = property class="MCListbox (strict)"(reference=w257) -> ("ItemNames"=w256:string[][])  [unwired: 1 in, 2 out]
                        n89 = Index Array(array=w256, index (col)=0 ("disabled index (col)")) -> (element=w254:string[])  [unwired: 1 in]
                        n90 = Unbundle By Name(w258) -> ("Column"=w248:i32, "Row"=w251:i32)
                        n91 = Array Size(array=w254) -> (size(s)=w250:i32)
                        n92 = Greater Or Equal To 0?(x=w251) -> (x >= 0?=w253:bool)
                        n93 = Less?(x=w251, y=w250) -> (x < y?=w249:bool)
                        n94 = Compound Arithmetic op=AND(w253, w249) -> (w252:bool)
                        n95 = case shown="True" w252 {
                          tunnel: w260 -> [_ w269]
                          tunnel: w259 -> [w264 w268]
                          tunnel: w258 -> [_ w267]
                          tunnel: [w263 w266] -> w247
                          tunnel: w248 -> [_ w265]
                          frame False {
                            n96 = property on="stepsRing" class="Ring (strict)"(error in=w264, "Visible"=FALSE) -> (error out=w263:errorcluster)  [unwired: 1 in, 1 out]
                          }
                          frame True {
                            n97 = case shown="0, Default" w265 {
                              tunnel: w269 -> [w286 w307 _]
                              tunnel: w268 -> [w284 w306 w311]
                              tunnel: w267 -> [w281 w305 _]
                              tunnel: [w287 w291 w308] -> w266
                              frame 0, Default {
                                w276 = TRUE ("Visible")
                                n98 = property on="Property Node" class="MCListbox (strict)"(reference=w286, error in=w284, "ActiveCell"=w281) -> (error out=w285:errorcluster, "ActiveCellPos"=w272:T11, "CellSize"=w275:T12, "CellFont"=w283:T21, "ItemNames"=w282:string[][])  [unwired: 1 out]
                                n99 = Unbundle By Name(w281) -> ("Row"=w280:i32)
                                n100 = Add(x=w272, y=T11 {"Left"=21, "Top"=0}) -> (x+y=w271:T11)
                                n101 = Subtract(x=w275, y=T12 {"Width"=21, "Height"=0}) -> (x-y=w273:T12)
                                n102 = Index Array(array=w282, index (row)=w280, index (col)=0 ("disabled index (col)")) -> (element=w278:string)
                                n103 = control-ref of="stepName"() -> (w288:refnum<vi>)
                                n104 = property on="Property Node" class="Str"(reference=w288, error in=w285, "Position"=w271, "Text.Size"=w273, "Text.Font"=w283, "Visible"=w276, "Key Focus"=w276, "Value"=w278) -> (error out=w287:errorcluster)  [unwired: 1 out]
                                n105 = property on="stepsRing" class="Ring (strict)"("Visible"=FALSE) -> ()  [unwired: 2 in, 2 out]
                              }
                              frame 1..3 {
                                w297 = TRUE ("Visible")
                                n106 = property on="Property Node" class="MCListbox (strict)"(reference=w307, error in=w306, "ActiveCell"=w305) -> (error out=w304:errorcluster, "ActiveCellPos"=w302:T11, "CellSize"=w300:T12, "CellFont"=w301:T21, "ItemNames"=w296:string[][])  [unwired: 1 out]
                                n107 = Index Array(array=w296, index (col)=0 ("disabled index (col)")) -> (element=w294:string[])  [unwired: 1 in]
                                n108 = Subtract(x=w300, y=T12 {"Width"=21, "Height"=0} ("x")) -> (x-y=w299:T12)
                                n109 = Build Array (concatenate)(string[] ["Next", "End", "--------------"], w294) -> (w292:string[])
                                n110 = control-ref of="stepsRing"() -> (w303:refnum<vi>)
                                n111 = property on="Property Node" class="Ring (strict)"(reference=w303, error in=w304, "Position"=w302, "RingText.Size"=w299, "RingText.Font"=w301, "Visible"=w297, "Key Focus"=w297, "Strings []"=w292, "Disabled Items []"=i32[] [2]) -> (error out=w291:errorcluster)  [unwired: 1 out]
                                n112 = property on="stepName" class="Str"("Visible"=FALSE) -> ()  [unwired: 2 in, 2 out]
                              }
                              frame 4 {
                                n113 = property on="stepsRing" class="Ring (strict)"(error in=w311, "Visible"=FALSE) -> (error out=w309:errorcluster)  [unwired: 1 in, 1 out]
                                n114 = property on="stepName" class="Str"(error in=w309, "Visible"=FALSE) -> (error out=w308:errorcluster)  [unwired: 1 in, 1 out]
                              }
                            }
                          }
                        }
                      }
                    }
                  }
                  frame Enabled {
                    n115 = property on="stepsRing" class="Ring (strict)"("Visible"=FALSE) -> (error out=w316:errorcluster)  [unwired: 2 in, 1 out]
                    n116 = property on="stepName" class="Str"(error in=w316, "Visible"=FALSE) -> (error out=w313:errorcluster)  [unwired: 1 in, 1 out]
                  }
                }
                n117 = Enqueue Element(queue=w236, element="System: Event User Handler") -> (queue out=w235:refnum<queue>)  [unwired: 2 in, 2 out]
              }
              event "Sequence List": Double Click {
                # "Button 1 = Left click"
                n118 = event-data() -> ("Button"=w317:u16, "CtlRef"=w319:refnum<vi>, "Coords"=w320:T20)  [unwired: 1 in, 1 out]
                n119 = case shown="1" w317 {
                  tunnel: w320 -> [_ w344]
                  tunnel: w319 -> [_ w341]
                  tunnel: [w326 w331] -> w318
                  frame 2, Default {
                    n120 = property on="stepsRing" class="Ring (strict)"("Visible"=FALSE) -> (error out=w328:errorcluster)  [unwired: 2 in, 1 out]
                    n121 = property on="stepName" class="Str"(error in=w328, "Visible"=FALSE) -> (error out=w326:errorcluster)  [unwired: 1 in, 1 out]
                  }
                  frame 1 {
                    n122 = invoke class="MCListbox (strict)" method="Point To Row Column"(reference=w341, "Point"=w344) -> (reference out=w343:refnum<vi>, error out=w342:errorcluster, "CellPosition"=w330:T2)  [unwired: 5 in, 4 out]
                    n123 = property class="MCListbox (strict)"(reference=w341) -> ("ItemNames"=w340:string[][])  [unwired: 1 in, 2 out]
                    n124 = Index Array(array=w340, index (col)=0 ("disabled index (col)")) -> (element=w338:string[])  [unwired: 1 in]
                    n125 = Unbundle By Name(w330) -> ("Column"=w332:i32, "Row"=w335:i32)
                    n126 = local write "Cell Position"(w330) -> ()
                    n127 = Array Size(array=w338) -> (size(s)=w334:i32)
                    n128 = Greater Or Equal To 0?(x=w335) -> (x >= 0?=w337:bool)
                    n129 = Less?(x=w335, y=w334) -> (x < y?=w333:bool)
                    n130 = Compound Arithmetic op=AND(w337, w333) -> (w336:bool)
                    n131 = case shown="True" w336 {
                      tunnel: w343 -> [_ w352]
                      tunnel: w342 -> [w347 w351]
                      tunnel: w330 -> [_ w350]
                      tunnel: [w346 w349] -> w331
                      tunnel: w332 -> [_ w348]
                      frame False {
                        n132 = property on="stepsRing" class="Ring (strict)"(error in=w347, "Visible"=FALSE) -> (error out=w346:errorcluster)  [unwired: 1 in, 1 out]
                      }
                      frame True {
                        n133 = case shown="1..3" w348 {
                          tunnel: w352 -> [w369 w397 _]
                          tunnel: w351 -> [w367 w396 w401]
                          tunnel: w350 -> [w364 w380 _]
                          tunnel: [w370 w384 w398] -> w349
                          frame 0, Default {
                            w359 = TRUE ("Visible")
                            n134 = property on="Property Node" class="MCListbox (strict)"(reference=w369, error in=w367, "ActiveCell"=w364) -> (error out=w368:errorcluster, "ActiveCellPos"=w355:T11, "CellSize"=w358:T12, "CellFont"=w366:T21, "ItemNames"=w365:string[][])  [unwired: 1 out]
                            n135 = Unbundle By Name(w364) -> ("Row"=w363:i32)
                            n136 = Add(x=w355, y=T11 {"Left"=21, "Top"=0}) -> (x+y=w354:T11)
                            n137 = Subtract(x=w358, y=T12 {"Width"=21, "Height"=0}) -> (x-y=w356:T12)
                            n138 = Index Array(array=w365, index (row)=w363, index (col)=0 ("disabled index (col)")) -> (element=w361:string)
                            n139 = control-ref of="stepName"() -> (w371:refnum<vi>)
                            n140 = property on="Property Node" class="Str"(reference=w371, error in=w368, "Position"=w354, "Text.Size"=w356, "Text.Font"=w366, "Visible"=w359, "Key Focus"=w359, "Value"=w361) -> (error out=w370:errorcluster)  [unwired: 1 out]
                            n141 = property on="stepsRing" class="Ring (strict)"("Visible"=FALSE) -> ()  [unwired: 2 in, 2 out]
                          }
                          frame 1..3 {
                            w388 = TRUE ("Visible")
                            n142 = property on="Property Node" class="MCListbox (strict)"(reference=w397, error in=w396, "ActiveCell"=w380) -> (error out=w395:errorcluster, "ActiveCellPos"=w393:T11, "CellSize"=w391:T12, "CellFont"=w392:T21, "ItemNames"=w381:string[][])  [unwired: 1 out]
                            n143 = Unbundle(w380) -> ("Row"=w379:i32, "Column"=w378:i32)
                            n144 = Index Array(array=w381, index (row)=w379, index (col)=w378) -> (element=w376:string)
                            n145 = Index Array(array=w381, index (col)=0 ("disabled index (col)")) -> (element=w386:string[])  [unwired: 1 in]
                            n146 = Subtract(x=w391, y=T12 {"Width"=21, "Height"=0} ("x")) -> (x-y=w390:T12)
                            n147 = Build Array (concatenate)(string[] ["Next", "End", "--------------"], w386) -> (w377:string[])
                            n148 = call "Search Unsorted 1D Array.vim"("element"=w376, "unsorted 1D array"=w377) -> ("index of element"=w374:i32)  [unwired: 9 in]
                            n149 = Greater Or Equal To 0?(x=w374) -> (x >= 0?=w375:bool)
                            n150 = control-ref of="stepsRing"() -> (w394:refnum<vi>)
                            n151 = Select(t=w374, s=w375, f=0) -> (s? t:f=w373:i32)
                            n152 = property on="stepName" class="Str"("Visible"=FALSE) -> ()  [unwired: 2 in, 2 out]
                            n153 = property on="Property Node" class="Ring (strict)"(reference=w394, error in=w395, "Position"=w393, "RingText.Size"=w390, "RingText.Font"=w392, "Visible"=w388, "Key Focus"=w388, "Strings []"=w377, "Disabled Items []"=i32[] [2], "Value"=w373) -> (error out=w384:errorcluster)  [unwired: 1 out]
                          }
                          frame 4 {
                            n154 = property on="stepsRing" class="Ring (strict)"(error in=w401, "Visible"=FALSE) -> (error out=w399:errorcluster)  [unwired: 1 in, 1 out]
                            n155 = property on="stepName" class="Str"(error in=w399, "Visible"=FALSE) -> (error out=w398:errorcluster)  [unwired: 1 in, 1 out]
                          }
                        }
                      }
                    }
                  }
                }
                n156 = Enqueue Element(queue=w323, element="System: Event User Handler") -> (queue out=w322:refnum<queue>)  [unwired: 2 in, 2 out]
              }
              event "stepName": Value Change {
                w407 = 0  # Step column
                n157 = event-data() -> ("NewVal"=w410:string)  [unwired: 1 in]
                n158 = local read "Cell Position"() -> (w409:T2)
                n159 = property on="Sequence List" class="MCListbox (strict)"() -> (error out=w412:errorcluster, "ItemNames"=w413:string[][])  [unwired: 2 in, 1 out]
                n160 = Unbundle(w409) -> ("Row"=w408:i32)  [unwired: 1 out]
                n161 = Replace Array Subset(array=w413, new element=w410, index (row)=w408, index (col)=w407) -> (w406:string[][])
                n162 = property on="Sequence List" class="MCListbox (strict)"(error in=w412, "ItemNames"=w406) -> (error out=w411:errorcluster)  [unwired: 1 in, 1 out]
                n163 = Enqueue Element(queue=w404, element="System: Event User Handler") -> (queue out=w405:refnum<queue>)  [unwired: 2 in, 2 out]
              }
              event "stepsRing": Value Change {
                n164 = event-data() -> ("CtlRef"=w420:refnum<vi>, "NewVal"=w418:u16)  [unwired: 1 in]
                n165 = property class="Ring (strict)"(reference=w420) -> (error out=w416:errorcluster, "Strings []"=w419:string[])  [unwired: 1 in, 1 out]
                n166 = Index Array(array=w419, index=w418) -> (element=w417:string)
                n167 = property on="Sequence List" class="MCListbox (strict)"(error in=w416) -> (error out=w429:errorcluster, "ItemNames"=w430:string[][])  [unwired: 1 in, 1 out]
                n168 = local read "Cell Position"() -> (w427:T2)
                n169 = Unbundle(w427) -> ("Row"=w422:i32, "Column"=w421:i32)
                n170 = Replace Array Subset(array=w430, new element=w417, index (row)=w422, index (col)=w421) -> (w426:string[][])
                n171 = property on="Sequence List" class="MCListbox (strict)"(error in=w429, "ItemNames"=w426) -> (error out=w428:errorcluster)  [unwired: 1 in, 1 out]
                n172 = Enqueue Element(queue=w424, element="System: Event User Handler") -> (queue out=w425:refnum<queue>)  [unwired: 2 in, 2 out]
              }
              event Timeout {
                n173 = event-data() -> ()  [unwired: 1 in, 3 out]
              }
            }
          }
          frame "System:Start" {
            # "Exec Mode\n1.) RUN -- Call by main program to run production\n2.) DEBUG -- VI Run it self in TOP level\n3.) OPEN VI -- Open front panel and block diagram of subVI\n4.) EDIT -- Run VI with allow user to edit criteria ,and sequence"
            # "If not run top level then use execMode from configure"
            # "Do not modify"
            n174 = control-ref of="This VI"() -> (w447:refnum<vi>)
            n175 = property class="VI"(reference=w447) -> (error out=w451:errorcluster, "Exec.State"=w453:T13)  [unwired: 1 in, 1 out]
            n176 = Unbundle By Name(w438) -> ("testConfigCluster.execMode"=w444:T9)
            n177 = Equal?(x=T13."Run top level", y=w453) -> (x = y?=w446:bool)
            n178 = local write "Tab Control"(enum32{"Sequence", "Input", "Output"}."Sequence" ("Tab Control")) -> ()
            n179 = Not(x=w446) -> (.not. x?=w445:bool)
            n180 = Select(t=w444, s=w445, f=__TEST__STEP__VAR__UI__EXEC__MODE__."Debug") -> (s? t:f=w437:T9)
            n181 = Bundle By Name(cluster=w438, "testConfigCluster.execMode"=w437) -> (w439:T4)
            n182 = case shown="\"Run\"" w437 {
              tunnel: w451 -> [_ _]
              tunnel: w450 -> [w457 w466]
              tunnel: [w456 w465] -> w449
              tunnel: w442 -> [w455 w464]
              tunnel: [w455 w464] -> w441
              tunnel: [w454 w463] -> w440
              tunnel: w439 -> [w454 w463]
              frame "Run" {
                n183 = for {
                  tunnel: w457 -> [w461]
                  tunnel: [w460] -> w456
                  tunnel: string[] ["System: Initialize", "System: Initial UI", "System: Load sequence config file", "System: Begin-Process"] -> [w459] mode=indexing
                  n184 = Enqueue Element(queue=w461, element=w459) -> (queue out=w460:refnum<queue>)  [unwired: 2 in, 2 out]
                }
              }
              frame Default {
                n185 = for {
                  tunnel: w466 -> [w469]
                  tunnel: [w468] -> w465
                  tunnel: string[] ["System: Initialize", "System: Initial UI", "System: Load sequence config file", "System: Event User Handler"] -> [w467] mode=indexing
                  n186 = Enqueue Element(queue=w469, element=w467) -> (queue out=w468:refnum<queue>)  [unwired: 2 in, 2 out]
                }
              }
            }
          }
          frame "System: Initialize" {
            # "Do not modify"
            n187 = Unbundle By Name(w472) -> ("testConfigCluster.execMode"=w471:T9)
            n188 = case shown="\"Run\"" w471 {
              tunnel: w472 -> [w476 w482]
              tunnel: [w476 w481] -> w475
              frame "Run" {
                # "Only \"Run\" mode will use reference control from VI who called this sequence module"
              }
              frame Default {
                n189 = control-ref of="testTable"() -> (w480:refnum<vi>)
                n190 = control-ref of="displayMsg"() -> (w479:refnum<vi>)
                n191 = local write "disMsg"(w479) -> ()
                n192 = local read "criteriaINI"() -> (w477:path)
                n193 = Bundle By Name(cluster=w482, "testConfigCluster.execMode"=__TEST__STEP__VAR__UI__EXEC__MODE__."Debug", "testConfigCluster.userControls.testTable"=w480, "testConfigCluster.userControls.dialog"=w479, "testConfigCluster.criteriaINI"=w477) -> (w481:T4)
              }
            }
          }
          frame "System: Initial UI" {
            w489 = 0 ("currentItem")
            # "Display criteria file path"
            # "Do not modify"
            n194 = Unbundle By Name(w484) -> ("testConfigCluster.execMode"=w492:T9)
            n195 = Unbundle By Name(w484) -> ("testConfigCluster.criteriaINI"=w485:path)
            n196 = property on="stepsRing" class="Ring (strict)"("Visible"=FALSE) -> (error out=w488:errorcluster)  [unwired: 2 in, 1 out]
            n197 = local write "totalSeqIndex"(w489) -> ()
            n198 = local write "currenIndex"(w489) -> ()
            n199 = local write "currentRetest"(w489) -> ()
            n200 = local write "criteriaINI"(w485) -> ()
            n201 = property on="stepName" class="Str"(error in=w488, "Visible"=FALSE) -> ()  [unwired: 1 in, 2 out]
            n202 = case shown="Default" w492 {
              tunnel: w484 -> [w502 w515]
              tunnel: [w497 w512] -> w494
              tunnel: [w502 w515] -> w493
              tunnel: w491 -> [w496 w507]
              tunnel: [w496 w507] -> w490
              frame "Run" {
                n203 = control-ref of="exitButton"() -> (w500:refnum<vi>)
                n204 = control-ref of="saveButton"() -> (w499:refnum<vi>)
                n205 = control-ref of="runButton"() -> (w498:refnum<vi>)
                n206 = Build Array(w500, w499, w498) -> (w501:refnum<vi>[])
                n207 = for {
                  tunnel: w501 -> [w505] mode=indexing
                  tunnel: [w504] -> w497
                  w503 = FALSE ("Value")
                  n208 = property class="Bool (strict)"(reference=w505, "Visible"=w503, "Value"=w503) -> (error out=w504:errorcluster)  [unwired: 1 in, 1 out]
                }
              }
              frame Default {
                n209 = Unbundle By Name(w515) -> ("testConfigCluster.userControls.dialog"=w514:refnum<vi>, "testConfigCluster"=w516:T8)
                n210 = Unbundle By Name(w515) -> ("stepData"=w518:T5)
                n211 = control-ref of="exitButton"() -> (w510:refnum<vi>)
                n212 = control-ref of="saveButton"() -> (w509:refnum<vi>)
                n213 = control-ref of="runButton"() -> (w508:refnum<vi>)
                n214 = Build Array(w510, w509, w508) -> (w511:refnum<vi>[])
                n215 = for {
                  tunnel: w511 -> [w525] mode=indexing
                  tunnel: [w523] -> w506
                  n216 = property class="Bool (strict)"(reference=w525, "Visible"=TRUE ("Value"), "Value"=FALSE) -> (error out=w523:errorcluster)  [unwired: 1 in, 1 out]
                }
                n217 = call <userlib>:"Tool.Update_Result_To_Table.vi"("Action"=__TABLE__ACTION__."Initial", "testConfigCluster"=w516, "error in (no error)"=w506, "seqDataIn"=w518) -> ("error out"=w520:errorcluster, "stepDutPara(Out)"=w517:T5)  [unwired: 6 in]
                n218 = call <userlib>:"Tool.Update_Result_To_Table.vi"("Action"=__TABLE__ACTION__."Clear", "testConfigCluster"=w516, "error in (no error)"=w520, "seqDataIn"=w517) -> ("error out"=w513:errorcluster)  [unwired: 6 in, 1 out]
                n219 = invoke class="Str" method="Reinit To Default"(reference=w514, error in=w513) -> (error out=w512:errorcluster)  [unwired: 1 in, 2 out]
              }
            }
          }
          frame "System: Load sequence config file" {
            # "Do not modify"
            n220 = control-ref of="This VI"() -> (w534:refnum<vi>)
            n221 = property class="VI"(reference=w534) -> ("Path"=w530:path)  [unwired: 1 in, 2 out]
            n222 = call <userlib>:"Get_variable_json_&_seq_csv_paths.vi"("seqPath"=w530) -> ("errorOut"=w528:errorcluster, "FoundAll ?"=w527:bool, "var&seqPaths[]"=w529:path[])  [unwired: 7 in, 1 out]
            n223 = for {
              shift-right: [w548] -> w533
              shift-left: w528 -> [w550]
              shift-right: [w544] -> w531
              shift-left: w532 -> [w545]
              tunnel: w529 -> [w543] mode=indexing
              tunnel: w527 -> [w539]
              n224 = call <vilib>:"Check if File or Folder Exists.vi"("error in (no error)"=w550, "path"=w543) -> ("error out"=w547:errorcluster, "file or folder exists?"=w541:bool, "dup path"=w538:path)  [unwired: 7 in]
              n225 = Empty String/Path?(string/path=w538) -> (empty?=w549:bool)
              n226 = Strip Path(path=w538) -> (name=w537:string)  [unwired: 1 out]
              n227 = Not(x=w549) -> (.not. x?=w542:bool)
              n228 = call <vilib>:"Clear Errors.vi"("error in (no error)"=w547) -> ("error out"=w546:errorcluster)  [unwired: 5 in, 1 out]
              n229 = Compound Arithmetic op=AND(w539, w542, w541) -> (w540:bool)
              n230 = case shown="\"sequence.csv\"" w537 {
                tunnel: w546 -> [w556 w587]
                tunnel: w538 -> [w553 w584]
                tunnel: [w555 w586] -> w548
                tunnel: w540 -> [w554 w585]
                tunnel: w545 -> [w552 w583]
                tunnel: [w551 w583] -> w544
                frame "variable.json", Default {
                  n231 = case shown="True" w554 {
                    tunnel: w556 -> [w558 w578]
                    tunnel: [w567 w573] -> w555
                    tunnel: w553 -> [w566 w571]
                    tunnel: w552 -> [w557 w570]
                    tunnel: [w557 w569] -> w551
                    frame False {
                      n232 = local read "userDef"() -> (w565:T3)
                      n233 = call <vilib>:"Flatten To JSON String.vi"("error in (no error)"=w558, "Variant"=w565) -> ("error out"=w559:errorcluster, "JSON String"=w560:string)  [unwired: 8 in]
                      n234 = Open/Create/Replace File(file path (use dialog)=w566, error in=w559, operation (0:open)=T10."create") -> (refnum out=w564:refnum<file>, error out=w562:errorcluster)  [unwired: 3 in, 1 out]
                      n235 = Write to Text File(file (use dialog)=w564, text=w560, error in=w562) -> (refnum out=w563:refnum<file>, error out=w561:errorcluster)  [unwired: 1 in, 1 out]
                      n236 = Close File(refnum=w563, error in=w561) -> (error out=w567:errorcluster)  [unwired: 1 out]
                    }
                    frame True {
                      n237 = Open/Create/Replace File(file path (use dialog)=w571, error in=w578, operation (0:open)=T10."open") -> (refnum out=w580:refnum<file>, error out=w582:errorcluster)  [unwired: 3 in, 1 out]
                      n238 = Read from Text File(file (use dialog)=w580, error in=w582) -> (refnum out=w579:refnum<file>, text=w575:string, error out=w581:errorcluster)  [unwired: 2 in, 1 out]
                      n239 = Close File(refnum=w579, error in=w581) -> (error out=w576:errorcluster)  [unwired: 1 out]
                      n240 = call <vilib>:"Unflatten From JSON String.vi"("Type and Defaults"=w570, "error in (no error)"=w576, "JSON String"=w575) -> ("error out"=w574:errorcluster, "Variant"=w572:variant)  [unwired: 7 in]
                      n241 = Variant To Data(error in=w574, type=w570, Variant=w572) -> (data=w569:T3, error out=w573:errorcluster)
                      n242 = local write "userDef"(w569) -> ()
                    }
                  }
                  n243 = local write "varFilePath"(w553) -> ()
                }
                frame "sequence.csv" {
                  n244 = case shown="True" w585 {
                    tunnel: w587 -> [w593 w608]
                    tunnel: [w591 w605] -> w586
                    tunnel: w584 -> [w588 w604]
                    frame False {
                      n245 = Open/Create/Replace File(file path (use dialog)=w588, error in=w593, operation (0:open)=T10."create") -> (refnum out=w595:refnum<file>, error out=w594:errorcluster)  [unwired: 3 in, 1 out]
                      n246 = Close File(refnum=w595, error in=w594) -> (error out=w592:errorcluster)  [unwired: 1 out]
                      n247 = property on="Sequence List" class="MCListbox (strict)"(error in=w592, "ItemNames"=string[][] [], "Value"=i32[] [] ("Sequence List")) -> (error out=w591:errorcluster)  [unwired: 1 in, 1 out]
                    }
                    frame True {
                      # "Delete first column (Enable flag)"
                      n248 = call-poly <vilib>:"Read Delimited Spreadsheet.vi"("file path (dialog if empty)"=w604, "error in (no error)"=w608, "delimiter (\\t)"="," ("delimiter (\\t)")) -> ("all rows"=w602:string[][], "error out"=w607:errorcluster)  [unwired: 7 in, 4 out]
                      n249 = Delete From Array(array=w602, index (col)=0 ("index (row)")) -> (deleted portion=w600:string[], array with subset deleted=w601:string[][])  [unwired: 2 in]
                      n250 = To Lower Case(string=w600) -> (all lower case string=w599:string[])
                      n251 = for {
                        tunnel: [w615] -> _ mode=indexing if=w612
                        tunnel: w599 -> [w614] mode=indexing
                        tunnel: [w609] -> w598 mode=indexing
                        i -> [w615]
                        n252 = Equal?(x=w614, y="enable") -> (x = y?=w612:bool)
                        n253 = Select(t=38, s=w612, f=37) -> (s? t:f=w609:i32)
                      }
                      n254 = property on="Sequence List" class="MCListbox (strict)"(error in=w607, "ItemNames"=w601, "ItemSyms"=w598, "Value"=i32[] [] ("Sequence List")) -> (error out=w605:errorcluster)  [unwired: 1 in, 1 out]
                    }
                  }
                  n255 = local write "seqFilePath"(w584) -> ()
                }
              }
            }
          }
          frame "System: Begin-Process" {
            # "Do not modify"
            n256 = property on="Sequence List" class="MCListbox (strict)"() -> ("ItemNames"=w618:string[][])  [unwired: 2 in, 2 out]
            n257 = Index Array(array=w618, index (col)=0 ("disabled index (col)")) -> (element=w621:string[])  [unwired: 1 in]
            n258 = Array Size(array=w621) -> (size(s)=w620:i32)
            n259 = local write "totalSeqIndex"(w620) -> ()
            n260 = local write "seqData[](Process)"(w618) -> ()
            n261 = local write "seqData[](Original)"(w618) -> ()
            n262 = Empty Array?(array=w618) -> (empty?=w625:bool)
            n263 = Select(t="System:End", s=w625, f="System:Pre-Process") -> (s? t:f=w626:string)
            n264 = Enqueue Element(queue=w628, element=w626) -> (queue out=w627:refnum<queue>)  [unwired: 2 in, 2 out]
          }
          frame "System:Pre-Process" {
            # "Get first index of arrays"
            # "Do not modify"
            n265 = local read "seqData[](Process)"() -> (w637:string[][])
            n266 = local read "currenIndex"() -> (w633:i32)
            n267 = Build Array(w633) -> (w635:i32[])
            n268 = Index Array(array=w637, index (row)=w633) -> (element=w636:string[])  [unwired: 1 in]
            n269 = property on="Sequence List" class="MCListbox (strict)"("Value"=w635) -> ("ItemSyms"=w634:i32[])  [unwired: 2 in, 2 out]
            n270 = Index Array(array=w634, index=w633) -> (element=w632:i32)
            n271 = Equal?(x=w632, y=38) -> (x = y?=w630:bool)
            n272 = case shown="False" w630 {
              tunnel: w642 -> [w664 w678]
              tunnel: [w663 w677] -> w641
              tunnel: [w662 w676] -> w640
              tunnel: w638 -> [w653 w673]
              tunnel: w636 -> [w651 w671]
              frame True {
                # "Clear data"
                n273 = Index Array(array=w651, index #1=T16."StepName", index #2=T16."PassTo", index #3=T16."FailTo", index #4=T16."ErrorTo", index #5=T15."Re-test") -> (element #1=w650:string, element #2=w656:string, element #3=w655:string, element #4=w654:string, element #5=w648:string)
                n274 = call <userlib>:"SEQ.Update_Seq_Var_Module.Init.vi"("mainVar"=w653) -> ("mainVarOut"=w661:T4)  [unwired: 2 in]
                n275 = Build Array (concatenate)(w650, string[] ["System:Post-Process:Check_Retest", "System:Post-Process:Update_Result"]) -> (w644:string[])
                n276 = Decimal String To Number(string=w648, default (0L)=u8 0 ("default (0 I32)")) -> (number=w647:u8)  [unwired: 1 in, 1 out]
                n277 = Reverse 1D Array(array=w644) -> (reversed array=w643:string[])
                n278 = Get Date/Time In Seconds() -> (seconds since 1Jan1904=w652:timestamp)
                n279 = for {
                  tunnel: w664 -> [w667]
                  tunnel: [w666] -> w663
                  tunnel: w643 -> [w665] mode=indexing
                  n280 = Enqueue Element At Opposite End(queue=w667, element=w665) -> (queue out=w666:refnum<queue>)  [unwired: 2 in, 2 out]
                }
                n281 = Bundle By Name(cluster=w661, "stepData.stepName"=w650, "stepData.passTo"=w656, "stepData.failTo"=w655, "stepData.errorTo"=w654, "stepData.retest"=w647, "stepData.startTime"=w652) -> (w662:T4)
              }
              frame False {
                # "Clear data"
                n282 = Index Array(array=w671, index=T16."StepName") -> (element=w670:string)
                n283 = call <userlib>:"SEQ.Update_Seq_Var_Module.Init.vi"("mainVar"=w673) -> ("mainVarOut"=w675:T4)  [unwired: 2 in]
                n284 = Get Date/Time In Seconds() -> (seconds since 1Jan1904=w672:timestamp)
                n285 = Bundle By Name(cluster=w675, "stepData.stepName"=w670, "stepData.startTime"=w672, "stepData.statusType"=__STEP__DATA__STATUS__TYPE__."SKIPPED") -> (w676:T4)
                n286 = Enqueue Element(queue=w678, element="System:Post-Process:Update_Result") -> (queue out=w677:refnum<queue>)  [unwired: 2 in, 2 out]
              }
            }
          }
          frame "System:Post-Process:Check_Retest" {
            # "Do not modify"
            n287 = Unbundle By Name(w683) -> ("stepData.statusType"=w684:T7)
            n288 = case shown="\"FAIL\"" w684 {
              tunnel: w683 -> [w689 w704]
              tunnel: [w688 w704] -> w682
              tunnel: w681 -> [w690 w703]
              tunnel: [w687 w703] -> w680
              frame "FAIL" {
                # "Retest over limit or have no Retest"
                n289 = Unbundle By Name(w689) -> ("stepData.retest"=w691:u8)
                n290 = local read "currentRetest"() -> (w692:u8)
                n291 = Greater Or Equal?(x=w692, y=w691) -> (x >= y?=w686:bool)
                n292 = case shown="False" w686 {
                  tunnel: w690 -> [w699 w701]
                  tunnel: w689 -> [w695 w702]
                  tunnel: [w695 w702] -> w688
                  tunnel: [w697 w701] -> w687
                  frame False {
                    # "Retest again"
                    n293 = local read "currentRetest"() -> (w694:u8)
                    n294 = Flush Queue(queue=w699) -> (queue out=w698:refnum<queue>)  [unwired: 1 in, 2 out]
                    n295 = Increment(x=w694) -> (x+1=w693:u8)
                    n296 = local write "currentRetest"(w693) -> ()
                    n297 = Enqueue Element(queue=w698, element="System:Pre-Process") -> (queue out=w697:refnum<queue>)  [unwired: 2 in, 2 out]
                  }
                  frame True {
                    # "Clear"
                    n298 = local write "currentRetest"(u8 0 ("currentItem")) -> ()
                  }
                }
              }
              frame Default {
              }
            }
          }
          frame "System:Post-Process:Update_Result" {
            # "Do not modify"
            n299 = Unbundle By Name(w707) -> ("stepData.statusType"=w708:T7)
            n300 = case shown="\"DONE\", \"PASS\"" w708 {
              tunnel: w707 -> [w718 w720 w722 _]
              tunnel: [w717 w719 w721 ""] -> w709
              frame "DONE", "PASS" {
                n301 = Unbundle By Name(w718) -> ("stepData.passTo"=w717:string)
              }
              frame "FAIL" {
                n302 = Unbundle By Name(w720) -> ("stepData.failTo"=w719:string)
              }
              frame "ERROR" {
                n303 = Unbundle By Name(w722) -> ("stepData.errorTo"=w721:string)
              }
              frame Default {
              }
            }
            n304 = local write "Tab Control"(enum32{"Sequence", "Input", "Output"}."Output" ("Tab Control")) -> ()
            n305 = local read "seqData[](Process)"() -> (w712:string[][])
            n306 = local read "currenIndex"() -> (w711:i32)
            n307 = call <userlib>:"ATMF.Get_Seq_Value_Index.vi"("seqData[]"=w712, "stepData.GoTo"=w709, "currenIndex"=w711) -> ("newIndex"=w710:i32)  [unwired: 8 in]
            n308 = call <userlib>:"SEQ.Append_Test_Result_To_Table.vi"("seqDataIn"=w707) -> ("seqDataOut"=w715:T4)  [unwired: 8 in, 2 out]
            n309 = case shown="-2" w710 {
              selector: w710 -> [w724 _ _]
              tunnel: w714 -> [w731 w734 w737]
              tunnel: [w730 w733 w736] -> w713
              frame Default {
                # "If new index more than total index size then finish testing"
                n310 = local read "totalSeqIndex"() -> (w726:i32)
                n311 = local write "currenIndex"(w724) -> ()
                n312 = Greater Or Equal?(x=w724, y=w726) -> (x >= y?=w725:bool)
                n313 = Select(t="System:End" ("element"), s=w725, f="System:Pre-Process" ("element")) -> (s? t:f=w727:string)
                n314 = Enqueue Element(queue=w731, element=w727) -> (queue out=w730:refnum<queue>)  [unwired: 2 in, 2 out]
              }
              frame -1 {
                # "Cannot find searched step name\n\nGo to end seq"
                n315 = Enqueue Element(queue=w734, element="System:End") -> (queue out=w733:refnum<queue>)  [unwired: 2 in, 2 out]
              }
              frame -2 {
                # "Go to end"
                n316 = Enqueue Element(queue=w737, element="System:End") -> (queue out=w736:refnum<queue>)  [unwired: 2 in, 2 out]
              }
            }
          }
          frame "System:End" {
            # "Do not modify"
            n317 = Unbundle By Name(w740) -> ("testConfigCluster.execMode"=w739:T9)
            n318 = case shown="Default" w739 {
              tunnel: [FALSE TRUE] -> w746
              tunnel: w745 -> [w752 w755]
              tunnel: [w752 w755] -> w744
              tunnel: w740 -> [w751 w754]
              tunnel: [w751 w754] -> w743
              tunnel: w742 -> [w748 w753]
              tunnel: [w749 w753] -> w741
              frame Default {
                n319 = Enqueue Element(queue=w748, element="System: Event User Handler") -> (queue out=w749:refnum<queue>)  [unwired: 2 in, 2 out]
              }
              frame "Run" {
              }
            }
          }
          frame Default {
            # "Do not modify"
            n320 = Concatenate Strings("Default case --> " ("message"), w763, "\nPlease check your test case is valid" ("string")) -> (w760:string)
            n321 = call "Display Message to User2"("Enable"=TRUE, "Message"=w760) -> ("error out"=w759:errorcluster)  [unwired: 8 in, 1 out]
          }
          frame "------------Developer Case------------" {
            # "Do not modify"
          }
          frame "init" {
            w788 = refnum<visa-resource-name> refnum ("VISA resource name")
            n322 = call "Read Ini.vi"("error in (no error)"=w790, "key"="DMM3058", "section"="Instrument") -> ("error out"=w789:errorcluster, "value"=w791:string)  [unwired: 7 in]
            n323 = call "Read Array Ini.vi"("error in (no error)"=w789, "Read_key"=string[] ["IO_Card", "Diagnostic_board"], "Section"="IO Card") -> ("error out"=w803:errorcluster, "Result_Value"=w802:string[])  [unwired: 7 in]
            n324 = call <userlib>:"SEQ.Update_Seq_Var_Module.Step_Name.vi"("Decription"="init", "mainVar"=w814, "Step Name"=w776) -> ("mainVarOut"=w810:T4)  [unwired: 4 in]
            n325 = call "Read Array Ini.vi"("error in (no error)"=w803, "Read_key"=string[] ["Control_BOX_LED", "UUT_LED", "Diagnostic_board"], "Section"="LED_right") -> ("error out"=w773:errorcluster, "Result_Value"=w798:string[])  [unwired: 7 in]
            n326 = Index Array(array=w802) -> (element #1=w801:string)  [unwired: 2 in, 1 out]
            n327 = Index Array(array=w798) -> (element #1=w797:string, element #2=w796:string, element #3=w772:string)  [unwired: 3 in]
            n328 = Type Cast(type=w788, x=w796) -> (*(type *) &x=w794:refnum<visa-resource-name>)
            n329 = Type Cast(type=w788, x=w797) -> (*(type *) &x=w795:refnum<visa-resource-name>)
            n330 = Type Cast(type=w788, x=w772) -> (*(type *) &x=w799:refnum<visa-resource-name>)
            n331 = Type Cast(type=w788, x=w791) -> (*(type *) &x=w782:refnum<visa-resource-name>)
            n332 = Type Cast(type=w788, x=w801) -> (*(type *) &x=w800:refnum<visa-resource-name>)
            n333 = call "DM3058 drive.vi"("Function Choose"=DM3058_Function_Choose."Init", "error in (no error)"=w773, "VISA resource name"=w782) -> ("error out"=w785:errorcluster, "VISA resource name out"=w786:refnum<visa-resource-name>)  [unwired: 6 in, 1 out]
            n334 = Bundle By Name(cluster=w808, "DMM3058"=w782, "IO_Card"=w800, "Diagnostic_board"=w799, "Control_BOX_LED"=w795, "UUT_LED"=w794) -> (w781:T1)
            n335 = call "DM3058 drive.vi"("Function Choose"=DM3058_Function_Choose."Config", "error in (no error)"=w785, "parameter"=T17 {"Reset (True)"=TRUE, "ID Query (True)"=FALSE, "Auto Range (T:Enable)"=FALSE, "Function (0: DC Volts)"=0, "Range Select"=enum."20V", "Absolute Resolution (0: 5.5 Rate:Slow)"=0}, "VISA resource name"=w786) -> ("error out"=w774:errorcluster)  [unwired: 5 in, 2 out]
            n336 = Format Into String(format string="%s", w776) -> (resulting string=w778:string)  [unwired: 2 in, 1 out]
            n337 = local read "disMsg"() -> (w779:refnum<vi>)
            n338 = call <userlib>:"ATMF.Disaplay_Msg_Console.vi"("errorIn"=w774, "Message"=w778, "dialogIn"=w779) -> ("errorOut"=w780:errorcluster)  [unwired: 7 in, 1 out]
            n339 = call-poly <userlib>:"[Polymorphic] SEQ.Update_Seq_Var_Module.vi"("UUT Error"=w780, "System Error In"=w775, "seqDataIn"=w810) -> ("System Error Out"=w812:errorcluster, "seqDataOut"=w813:T4)  [unwired: 7 in]
          }
          frame "Set SW3 OFF" {
            # "Close SW3"
            n340 = Unbundle By Name(w822) -> ("IO_Card"=w829:refnum<visa-resource-name>)
            n341 = call <userlib>:"SEQ.Update_Seq_Var_Module.Step_Name.vi"("Decription"="Set SW3 OFF", "mainVar"=w821, "Step Name"=w820) -> ("mainVarOut"=w832:T4)  [unwired: 4 in]
            n342 = call "DCDC_Command.vi"("error in (no error)"=w824, "State"=FALSE, "Function Choose"=DCDC_Command."FCT_SW3", "VISA resource in"=w829) -> ("error out"=w826:errorcluster)  [unwired: 4 in, 3 out]
            n343 = Format Into String(format string="%s", w820) -> (resulting string=w828:string)  [unwired: 2 in, 1 out]
            n344 = local read "disMsg"() -> (w816:refnum<vi>)
            n345 = call <userlib>:"ATMF.Disaplay_Msg_Console.vi"("errorIn"=w826, "Message"=w828, "dialogIn"=w816) -> ("errorOut"=w827:errorcluster)  [unwired: 7 in, 1 out]
            n346 = call-poly <userlib>:"[Polymorphic] SEQ.Update_Seq_Var_Module.vi"("UUT Error"=w827, "System Error In"=w819, "seqDataIn"=w832) -> ("System Error Out"=w817:errorcluster, "seqDataOut"=w818:T4)  [unwired: 7 in]
          }
          frame "Measure L1 ON" {
            n347 = Unbundle By Name(w849) -> ("Control_BOX_LED"=w839:refnum<visa-resource-name>)
            n348 = call <userlib>:"SEQ.Update_Seq_Var_Module.Step_Name.vi"("Decription"="Measure L1 ON", "mainVar"=w855, "Step Name"=w843) -> ("mainVarOut"=w850:T4)  [unwired: 4 in]
            n349 = Unbundle By Name(w851) -> ()  [unwired: 2 out]
            n350 = call "LED_Command.vi"("L lower limit"=25, "Hue lower limit"=65, "L upper limit"=70, "Hue upper limit"=150, "error in (no error)"=w842, "channel"="1", "VISA resource in"=w839) -> ("error out"=w841:errorcluster, "Result"=w840:bool)  [unwired: 1 in, 2 out]
            n351 = Format Into String(format string="%s    %s", w843, w840) -> (resulting string=w847:string)  [unwired: 2 in, 1 out]
            n352 = local read "disMsg"() -> (w848:refnum<vi>)
            n353 = call <userlib>:"ATMF.Disaplay_Msg_Console.vi"("errorIn"=w841, "Message"=w847, "dialogIn"=w848) -> ("errorOut"=w845:errorcluster)  [unwired: 7 in, 1 out]
            n354 = call-poly <userlib>:"[Polymorphic] SEQ.Update_Seq_Var_Module.vi"("UUT Error"=w845, "System Error In"=w844, "value"=w840, "seqDataIn"=w850) -> ("System Error Out"=w853:errorcluster, "seqDataOut"=w854:T4)  [unwired: 6 in]
          }
          frame "Measure L3 ON" {
            n355 = Unbundle By Name(w872) -> ("Control_BOX_LED"=w862:refnum<visa-resource-name>)
            n356 = call <userlib>:"SEQ.Update_Seq_Var_Module.Step_Name.vi"("Decription"="Measure L3 ON", "mainVar"=w878, "Step Name"=w866) -> ("mainVarOut"=w873:T4)  [unwired: 4 in]
            n357 = Unbundle By Name(w874) -> ()  [unwired: 2 out]
            n358 = call "LED_Command.vi"("L lower limit"=25, "Hue lower limit"=65, "L upper limit"=70, "Hue upper limit"=150, "error in (no error)"=w863, "channel"="3", "VISA resource in"=w862) -> ("error out"=w864:errorcluster, "Result"=w861:bool)  [unwired: 1 in, 2 out]
            n359 = Format Into String(format string="%s    %s", w866, w861) -> (resulting string=w869:string)  [unwired: 2 in, 1 out]
            n360 = local read "disMsg"() -> (w870:refnum<vi>)
            n361 = call <userlib>:"ATMF.Disaplay_Msg_Console.vi"("errorIn"=w864, "Message"=w869, "dialogIn"=w870) -> ("errorOut"=w867:errorcluster)  [unwired: 7 in, 1 out]
            n362 = call-poly <userlib>:"[Polymorphic] SEQ.Update_Seq_Var_Module.vi"("UUT Error"=w867, "System Error In"=w871, "value"=w861, "seqDataIn"=w873) -> ("System Error Out"=w876:errorcluster, "seqDataOut"=w877:T4)  [unwired: 6 in]
          }
          frame "Measure UUT D3 ON" {
            n363 = Unbundle By Name(w895) -> ("UUT_LED"=w884:refnum<visa-resource-name>)
            n364 = call <userlib>:"SEQ.Update_Seq_Var_Module.Step_Name.vi"("Decription"=" Measure UUT D3 ON ", "mainVar"=w901, "Step Name"=w890) -> ("mainVarOut"=w896:T4)  [unwired: 4 in]
            n365 = Unbundle By Name(w897) -> ()  [unwired: 2 out]
            n366 = call "LED_Command.vi"("L lower limit"=25, "Hue lower limit"=65, "L upper limit"=70, "Hue upper limit"=150, "error in (no error)"=w885, "channel"="1", "VISA resource in"=w884) -> ("error out"=w886:errorcluster, "Result"=w887:bool)  [unwired: 1 in, 2 out]
            n367 = Format Into String(format string="%s    %s", w890, w887) -> (resulting string=w893:string)  [unwired: 2 in, 1 out]
            n368 = local read "disMsg"() -> (w894:refnum<vi>)
            n369 = call <userlib>:"ATMF.Disaplay_Msg_Console.vi"("errorIn"=w886, "Message"=w893, "dialogIn"=w894) -> ("errorOut"=w891:errorcluster)  [unwired: 7 in, 1 out]
            n370 = call-poly <userlib>:"[Polymorphic] SEQ.Update_Seq_Var_Module.vi"("UUT Error"=w891, "System Error In"=w889, "value"=w887, "seqDataIn"=w896) -> ("System Error Out"=w899:errorcluster, "seqDataOut"=w900:T4)  [unwired: 6 in]
          }
          frame "Measure UUT D5 ON" {
            n371 = Unbundle By Name(w918) -> ("UUT_LED"=w908:refnum<visa-resource-name>)
            n372 = call <userlib>:"SEQ.Update_Seq_Var_Module.Step_Name.vi"("Decription"="Measure UUT D5 ON", "mainVar"=w924, "Step Name"=w912) -> ("mainVarOut"=w919:T4)  [unwired: 4 in]
            n373 = Unbundle By Name(w920) -> ()  [unwired: 2 out]
            n374 = call "LED_Command.vi"("L lower limit"=25, "Hue lower limit"=65, "L upper limit"=70, "Hue upper limit"=150, "error in (no error)"=w909, "channel"="3", "VISA resource in"=w908) -> ("error out"=w910:errorcluster, "Result"=w907:bool)  [unwired: 1 in, 2 out]
            n375 = Format Into String(format string="%s    %s", w912, w907) -> (resulting string=w915:string)  [unwired: 2 in, 1 out]
            n376 = local read "disMsg"() -> (w916:refnum<vi>)
            n377 = call <userlib>:"ATMF.Disaplay_Msg_Console.vi"("errorIn"=w910, "Message"=w915, "dialogIn"=w916) -> ("errorOut"=w913:errorcluster)  [unwired: 7 in, 1 out]
            n378 = call-poly <userlib>:"[Polymorphic] SEQ.Update_Seq_Var_Module.vi"("UUT Error"=w913, "System Error In"=w917, "value"=w907, "seqDataIn"=w919) -> ("System Error Out"=w922:errorcluster, "seqDataOut"=w923:T4)  [unwired: 6 in]
          }
          frame "Measure UUT D6 ON" {
            n379 = Unbundle By Name(w941) -> ("UUT_LED"=w930:refnum<visa-resource-name>)
            n380 = call <userlib>:"SEQ.Update_Seq_Var_Module.Step_Name.vi"("Decription"="Measure UUT D6 ON", "mainVar"=w947, "Step Name"=w935) -> ("mainVarOut"=w942:T4)  [unwired: 4 in]
            n381 = Unbundle By Name(w943) -> ()  [unwired: 2 out]
            n382 = call "LED_Command.vi"("L lower limit"=25, "Hue lower limit"=65, "L upper limit"=70, "Hue upper limit"=150, "error in (no error)"=w931, "channel"="4", "VISA resource in"=w930) -> ("error out"=w932:errorcluster, "Result"=w933:bool)  [unwired: 1 in, 2 out]
            n383 = Format Into String(format string="%s    %s", w935, w933) -> (resulting string=w938:string)  [unwired: 2 in, 1 out]
            n384 = local read "disMsg"() -> (w939:refnum<vi>)
            n385 = call <userlib>:"ATMF.Disaplay_Msg_Console.vi"("errorIn"=w932, "Message"=w938, "dialogIn"=w939) -> ("errorOut"=w936:errorcluster)  [unwired: 7 in, 1 out]
            n386 = call-poly <userlib>:"[Polymorphic] SEQ.Update_Seq_Var_Module.vi"("UUT Error"=w936, "System Error In"=w940, "value"=w933, "seqDataIn"=w942) -> ("System Error Out"=w945:errorcluster, "seqDataOut"=w946:T4)  [unwired: 6 in]
          }
          frame "Measure UUT D8 ON" {
            n387 = Unbundle By Name(w964) -> ("UUT_LED"=w953:refnum<visa-resource-name>)
            n388 = call <userlib>:"SEQ.Update_Seq_Var_Module.Step_Name.vi"("Decription"="Measure UUT D8 ON", "mainVar"=w970, "Step Name"=w959) -> ("mainVarOut"=w965:T4)  [unwired: 4 in]
            n389 = Unbundle By Name(w966) -> ()  [unwired: 2 out]
            n390 = call "LED_Command.vi"("L lower limit"=25, "Hue lower limit"=65, "L upper limit"=70, "Hue upper limit"=150, "error in (no error)"=w955, "channel"="6", "VISA resource in"=w953) -> ("error out"=w956:errorcluster, "Result"=w954:bool)  [unwired: 1 in, 2 out]
            n391 = Format Into String(format string="%s    %s", w959, w954) -> (resulting string=w962:string)  [unwired: 2 in, 1 out]
            n392 = local read "disMsg"() -> (w963:refnum<vi>)
            n393 = call <userlib>:"ATMF.Disaplay_Msg_Console.vi"("errorIn"=w956, "Message"=w962, "dialogIn"=w963) -> ("errorOut"=w960:errorcluster)  [unwired: 7 in, 1 out]
            n394 = call-poly <userlib>:"[Polymorphic] SEQ.Update_Seq_Var_Module.vi"("UUT Error"=w960, "System Error In"=w958, "value"=w954, "seqDataIn"=w965) -> ("System Error Out"=w968:errorcluster, "seqDataOut"=w969:T4)  [unwired: 6 in]
          }
          frame "Measure APOS UUT Voltages_SW3_OFF" {
            n395 = Unbundle By Name(w992) -> ("DMM3058"=w989:refnum<visa-resource-name>, "IO_Card"=w991:refnum<visa-resource-name>, "Diagnostic_board"=w974:refnum<visa-resource-name>)
            n396 = call <userlib>:"SEQ.Update_Seq_Var_Module.Step_Name.vi"("Decription"=" Measure APOS UUT Voltages_SW3_OFF", "mainVar"=w996, "Step Name"=w981) -> ("mainVarOut"=w976:T4)  [unwired: 4 in]
            n397 = Unbundle By Name(w988) -> ("APOS Max"=w973:dbl, "APOS Min"=w972:dbl)
            n398 = disable-structure shown="Enabled" {
              disable-tunnel: w991 -> [w1006 _]
              disable-tunnel: w990 -> [w1005 w1018]
              disable-tunnel: w989 -> [w1004 _]
              disable-tunnel: [w1001 w1017] -> w983
              disable-tunnel: [w1000 w1016] -> w978
              disable-tunnel: w974 -> [_ w1015]
              disable-tunnel: w973 -> [_ w1013]
              disable-tunnel: w972 -> [_ w1012]
              frame Disabled {
                w1002 = DCDC_Command."meas_UUT_APOS_voltage" ("Function Choose")
                n399 = call "DCDC_Command.vi"("error in (no error)"=w1005, "State"=TRUE, "Function Choose"=w1002, "VISA resource in"=w1006) -> ("error out"=w1003:errorcluster, "VISA resource out"=w1008:refnum<visa-resource-name>)  [unwired: 4 in, 2 out]
                n400 = call "Stall Data Flow.vim"("value in"=w1003, "milliseconds to wait"=u32 2000) -> ("value out"=w999:errorcluster)  [unwired: 1 out]
                n401 = call "DM3058 drive.vi"("Function Choose"=DM3058_Function_Choose."Measure", "error in (no error)"=w999, "VISA resource name"=w1004) -> ("error out"=w1007:errorcluster, "Measurement"=w1000:dbl)  [unwired: 6 in, 1 out]
                n402 = call "DCDC_Command.vi"("error in (no error)"=w1007, "State"=FALSE, "Function Choose"=w1002, "VISA resource in"=w1008) -> ("error out"=w1001:errorcluster)  [unwired: 4 in, 3 out]
              }
              frame Enabled {
                n403 = for {
                  N: 200 -> [_]
                  tunnel: [w1019] -> w1016
                  tunnel: w1015 -> [w1023]
                  shift-right: [w1024] -> w1017
                  shift-left: w1018 -> [w1025]
                  tunnel: w1013 -> [w1021]
                  tunnel: w1012 -> [w1020]
                  stop <- w1022 stop-if-true
                  n404 = call "UUT modules Read Temperature and Voltages.vi"("error in (no error)"=w1025, "VISA resource name"=w1023) -> ("error out"=w1024:errorcluster, "APOS_Voltage"=w1019:dbl)  [unwired: 3 in, 5 out]
                  n405 = In Range and Coerce(upper limit=w1021, x=w1019, lower limit=w1020) -> (In Range?=w1022:bool)  [unwired: 1 out]
                }
              }
            }
            n406 = Number To Fractional String(number=w973) -> (F-format string=w980:string)  [unwired: 3 in]
            n407 = Number To Fractional String(number=w972) -> (F-format string=w979:string)  [unwired: 3 in]
            n408 = call-poly <userlib>:"[Polymorphic] SEQ.Update_Seq_Var_Module.Set_Max_Min.vi"("stepData.min"=w979, "stepData.max"=w980, "seqDataIn"=w976) -> ("seqDataOut"=w975:T4)  [unwired: 8 in]
            n409 = Format Into String(format string="%s    %d", w981, w978) -> (resulting string=w986:string)  [unwired: 2 in, 1 out]
            n410 = local read "disMsg"() -> (w987:refnum<vi>)
            n411 = call <userlib>:"ATMF.Disaplay_Msg_Console.vi"("errorIn"=w983, "Message"=w986, "dialogIn"=w987) -> ("errorOut"=w984:errorcluster)  [unwired: 7 in, 1 out]
            n412 = call-poly <userlib>:"[Polymorphic] SEQ.Update_Seq_Var_Module.vi"("UUT Error"=w984, "System Error In"=w982, "value"=w978, "Unit"="V", "seqDataIn"=w975) -> ("System Error Out"=w994:errorcluster, "seqDataOut"=w993:T4)  [unwired: 5 in]
          }
          frame "Measure ANEG UUT Voltages_SW3_OFF" {
            n413 = Unbundle By Name(w1043) -> ("DMM3058"=w1045:refnum<visa-resource-name>, "IO_Card"=w1046:refnum<visa-resource-name>, "Diagnostic_board"=w1028:refnum<visa-resource-name>)
            n414 = call <userlib>:"SEQ.Update_Seq_Var_Module.Step_Name.vi"("Decription"="Measure ANEG UUT Voltages_SW3_OFF", "mainVar"=w1050, "Step Name"=w1036) -> ("mainVarOut"=w1032:T4)  [unwired: 4 in]
            n415 = Unbundle By Name(w1042) -> ("ANEG Max"=w1027:dbl, "ANEG Min"=w1026:dbl)
            n416 = disable-structure shown="Enabled" {
              disable-tunnel: w1046 -> [w1060 _]
              disable-tunnel: w1045 -> [w1059 _]
              disable-tunnel: w1044 -> [w1057 w1072]
              disable-tunnel: [w1055 w1071] -> w1037
              disable-tunnel: [w1054 w1069] -> w1030
              disable-tunnel: w1028 -> [_ w1070]
              disable-tunnel: w1027 -> [_ w1067]
              disable-tunnel: w1026 -> [_ w1066]
              frame Disabled {
                w1056 = DCDC_Command."meas_UUT_ANEG_voltage" ("Function Choose")
                n417 = call "DCDC_Command.vi"("error in (no error)"=w1057, "State"=TRUE, "Function Choose"=w1056, "VISA resource in"=w1060) -> ("error out"=w1058:errorcluster, "VISA resource out"=w1062:refnum<visa-resource-name>)  [unwired: 4 in, 2 out]
                n418 = call "Stall Data Flow.vim"("value in"=w1058, "milliseconds to wait"=u32 500) -> ("value out"=w1053:errorcluster)  [unwired: 1 out]
                n419 = call "DM3058 drive.vi"("Function Choose"=DM3058_Function_Choose."Measure", "error in (no error)"=w1053, "VISA resource name"=w1059) -> ("error out"=w1061:errorcluster, "Measurement"=w1054:dbl)  [unwired: 6 in, 1 out]
                n420 = call "DCDC_Command.vi"("error in (no error)"=w1061, "State"=FALSE, "Function Choose"=w1056, "VISA resource in"=w1062) -> ("error out"=w1055:errorcluster)  [unwired: 4 in, 3 out]
              }
              frame Enabled {
                n421 = for {
                  N: 200 -> [_]
                  tunnel: w1070 -> [w1077]
                  tunnel: [w1073] -> w1069
                  shift-right: [w1078] -> w1071
                  shift-left: w1072 -> [w1079]
                  tunnel: w1067 -> [w1075]
                  tunnel: w1066 -> [w1074]
                  stop <- w1076 stop-if-true
                  n422 = call "UUT modules Read Temperature and Voltages.vi"("error in (no error)"=w1079, "VISA resource name"=w1077) -> ("error out"=w1078:errorcluster, "ANEG_Voltage"=w1073:dbl)  [unwired: 3 in, 5 out]
                  n423 = In Range and Coerce(upper limit=w1075, x=w1073, lower limit=w1074) -> (In Range?=w1076:bool)  [unwired: 1 out]
                }
              }
            }
            n424 = Number To Fractional String(number=w1027) -> (F-format string=w1034:string)  [unwired: 3 in]
            n425 = Number To Fractional String(number=w1026) -> (F-format string=w1033:string)  [unwired: 3 in]
            n426 = call-poly <userlib>:"[Polymorphic] SEQ.Update_Seq_Var_Module.Set_Max_Min.vi"("stepData.min"=w1033, "stepData.max"=w1034, "seqDataIn"=w1032) -> ("seqDataOut"=w1031:T4)  [unwired: 8 in]
            n427 = Format Into String(format string="%s    %d", w1036, w1030) -> (resulting string=w1040:string)  [unwired: 2 in, 1 out]
            n428 = local read "disMsg"() -> (w1041:refnum<vi>)
            n429 = call <userlib>:"ATMF.Disaplay_Msg_Console.vi"("errorIn"=w1037, "Message"=w1040, "dialogIn"=w1041) -> ("errorOut"=w1038:errorcluster)  [unwired: 7 in, 1 out]
            n430 = call-poly <userlib>:"[Polymorphic] SEQ.Update_Seq_Var_Module.vi"("UUT Error"=w1038, "System Error In"=w1035, "value"=w1030, "Unit"="V", "seqDataIn"=w1031) -> ("System Error Out"=w1048:errorcluster, "seqDataOut"=w1047:T4)  [unwired: 5 in]
          }
          frame "Measure DPOS UUT Voltages_SW3_OFF" {
            n431 = Unbundle By Name(w1098) -> ("DMM3058"=w1097:refnum<visa-resource-name>, "IO_Card"=w1099:refnum<visa-resource-name>, "Diagnostic_board"=w1082:refnum<visa-resource-name>)
            n432 = call <userlib>:"SEQ.Update_Seq_Var_Module.Step_Name.vi"("Decription"=" Measure DPOS UUT Voltages_SW3_OFF", "mainVar"=w1104, "Step Name"=w1089) -> ("mainVarOut"=w1086:T4)  [unwired: 4 in]
            n433 = Unbundle By Name(w1096) -> ("DPOS Max"=w1081:dbl, "DPOS Min"=w1080:dbl)
            n434 = disable-structure shown="Enabled" {
              disable-tunnel: w1100 -> [w1110 w1124]
              disable-tunnel: w1099 -> [w1109 _]
              disable-tunnel: w1097 -> [w1108 _]
              disable-tunnel: [w1107 w1123] -> w1092
              disable-tunnel: [w1106 w1121] -> w1084
              disable-tunnel: w1082 -> [_ w1122]
              disable-tunnel: w1081 -> [_ w1119]
              disable-tunnel: w1080 -> [_ w1118]
              frame Disabled {
                w1111 = DCDC_Command."meas_UUT_APOS_voltage" ("Function Choose")
                n435 = call "DCDC_Command.vi"("error in (no error)"=w1110, "State"=TRUE, "Function Choose"=w1111, "VISA resource in"=w1109) -> ("error out"=w1112:errorcluster, "VISA resource out"=w1114:refnum<visa-resource-name>)  [unwired: 4 in, 2 out]
                n436 = call "DM3058 drive.vi"("Function Choose"=DM3058_Function_Choose."Measure", "error in (no error)"=w1112, "VISA resource name"=w1108) -> ("error out"=w1113:errorcluster, "Measurement"=w1106:dbl)  [unwired: 6 in, 1 out]
                n437 = call "DCDC_Command.vi"("error in (no error)"=w1113, "State"=FALSE, "Function Choose"=w1111, "VISA resource in"=w1114) -> ("error out"=w1107:errorcluster)  [unwired: 4 in, 3 out]
              }
              frame Enabled {
                n438 = for {
                  N: 200 -> [_]
                  tunnel: w1122 -> [w1129]
                  tunnel: [w1125] -> w1121
                  shift-right: [w1130] -> w1123
                  shift-left: w1124 -> [w1131]
                  tunnel: w1119 -> [w1127]
                  tunnel: w1118 -> [w1126]
                  stop <- w1128 stop-if-true
                  n439 = call "UUT modules Read Temperature and Voltages.vi"("error in (no error)"=w1131, "VISA resource name"=w1129) -> ("error out"=w1130:errorcluster, "DPOS_Voltage"=w1125:dbl)  [unwired: 3 in, 5 out]
                  n440 = In Range and Coerce(upper limit=w1127, x=w1125, lower limit=w1126) -> (In Range?=w1128:bool)  [unwired: 1 out]
                }
              }
            }
            n441 = Number To Fractional String(number=w1081) -> (F-format string=w1088:string)  [unwired: 3 in]
            n442 = Number To Fractional String(number=w1080) -> (F-format string=w1087:string)  [unwired: 3 in]
            n443 = call-poly <userlib>:"[Polymorphic] SEQ.Update_Seq_Var_Module.Set_Max_Min.vi"("stepData.min"=w1087, "stepData.max"=w1088, "seqDataIn"=w1086) -> ("seqDataOut"=w1085:T4)  [unwired: 8 in]
            n444 = Format Into String(format string="%s    %d", w1089, w1084) -> (resulting string=w1094:string)  [unwired: 2 in, 1 out]
            n445 = local read "disMsg"() -> (w1095:refnum<vi>)
            n446 = call <userlib>:"ATMF.Disaplay_Msg_Console.vi"("errorIn"=w1092, "Message"=w1094, "dialogIn"=w1095) -> ("errorOut"=w1093:errorcluster)  [unwired: 7 in, 1 out]
            n447 = call-poly <userlib>:"[Polymorphic] SEQ.Update_Seq_Var_Module.vi"("UUT Error"=w1093, "System Error In"=w1091, "value"=w1084, "Unit"="V", "seqDataIn"=w1085) -> ("System Error Out"=w1102:errorcluster, "seqDataOut"=w1101:T4)  [unwired: 5 in]
          }
          frame "Power Off" {
            # "Close SW1"
            # "Close PSU"
            n448 = Unbundle By Name(w1134) -> ("IO_Card"=w1133:refnum<visa-resource-name>)
            n449 = call "DCDC_Command.vi"("error in (no error)"=w1141, "State"=FALSE, "Function Choose"=DCDC_Command."FCT_SW1", "VISA resource in"=w1133) -> ("error out"=w1138:errorcluster, "VISA resource out"=w1132:refnum<visa-resource-name>)  [unwired: 4 in, 2 out]
            n450 = call <userlib>:"SEQ.Update_Seq_Var_Module.Step_Name.vi"("Decription"="Power Off", "mainVar"=w1148, "Step Name"=w1149) -> ("mainVarOut"=w1150:T4)  [unwired: 4 in]
            n451 = call "Stall Data Flow.vim"("value in"=w1138, "milliseconds to wait"=u32 500) -> ("value out"=w1136:errorcluster)  [unwired: 1 out]
            n452 = call "DCDC_Command.vi"("error in (no error)"=w1136, "State"=FALSE, "Function Choose"=DCDC_Command."UUT_FCT_power_SW", "VISA resource in"=w1132) -> ("error out"=w1137:errorcluster)  [unwired: 4 in, 3 out]
            n453 = call-poly <userlib>:"[Polymorphic] SEQ.Update_Seq_Var_Module.vi"("System Error In"=w1137, "seqDataIn"=w1150) -> ("System Error Out"=w1145:errorcluster, "seqDataOut"=w1144:T4)  [unwired: 8 in]
          }
        }
      }
      frame Error {
        # "Bypass system error out to main program"
        n454 = Flush Queue(queue=w1155) -> (queue out=w1157:refnum<queue>)  [unwired: 1 in, 2 out]
        n455 = Enqueue Element(queue=w1157, element="End") -> (queue out=w1158:refnum<queue>)  [unwired: 2 in, 2 out]
      }
    }
    n456 = call <userlib>:"SEQ.Post_Process.CheckSeqDone&StopEvent.vi"("sysErrorIn(noError)"=w26, "mainVar"=w28) -> ("sysErrorIOut"=w25:errorcluster, "userStop??"=w24:bool, "mainVarOut"=w27:T4)  [unwired: 7 in]
    n457 = Or(x=w24, y=w23) -> (x .or. y?=w22:bool)
  }
  "System Error Out" <- w11
  n458 = Unbundle By Name(w5) -> ("testConfigCluster"=w4:T8)
  n459 = Flush Queue(queue=w16) -> (queue out=w18:refnum<queue>, error out=w12:errorcluster)  [unwired: 1 in, 1 out]
  n460 = Release Queue(queue=w18, error in (no error)=w12) -> (error out=w13:errorcluster)  [unwired: 1 in, 2 out]
  n461 = call <vilib>:"Clear Errors.vi"("error in (no error)"=w13) -> ()  [unwired: 5 in, 2 out]
  n462 = To Variant(anything=w4) -> (Variant=→"variantOut":variant)
